vi "FFT_DAS_GUI(2).vi"() -> ()   [LabVIEW 2010]
doc: "<b>LITVC - ?????????????????????</b>\n\nMeasures, graphs and logs the data from the LITVC cRIO Chassis. Samples 12 analog channels of raw at kilohertz speeds, and controls starting of test data runs, with triggered control of the appropriate solenoid valves . \n\nSystem scaling and other constants are loaded from the \"LITVC_CFG.TXT\" text file at startup. (The order of the lines must remain the same. ) The Operator must supply a data file path and name at startup. This defaults on the cRIO Controller to: \"C:\\Data\". The software then starts data acquisition and logging, as indicated by the blinking green \"Active\" LED.\n\nPressing \"CAL\" after start will calibrate the system to the cross section of the wire rope.\nTo stop the acquisition, press the Stop button in the upper right. This allows the operator to look at the graphs, error indicators, etc on the status tab.\nTo Exit, press the EXIT button on the Status tab.\n\nVersion 1.0.0:\n 1. Initial version\n\n2010_09_30 Michael Ashe\nmichael.ashe@aztera.com\nmichael.ashe@imaginatics.net\n(860) 961-0876 (Cell)"
uses:
  Common/Controls/GUI_Buttons_23x22_W2K.llb/FileGroup_1.ctl
  Common/Controls/GUI_Buttons_23x22_W2K.llb/New.ctl
  Common/Controls/GUI_Buttons_23x22_W2K.llb/Open.ctl
  Common/Controls/GUI_Buttons_23x22_W2K.llb/Save.ctl
  Common/Controls/GUI_Buttons_23x22_W2K.llb/EditGroup_1.ctl
  Common/Controls/GUI_Buttons_23x22_W2K.llb/Cut.ctl
  Common/Controls/GUI_Buttons_23x22_W2K.llb/Copy.ctl
  Common/Controls/GUI_Buttons_23x22_W2K.llb/Paste.ctl
  Common/Controls/GUI_Buttons_23x22_W2K.llb/Delete1.ctl
  Common/Controls/GUI_Buttons_23x22_W2K.llb/MacroPlay.ctl
  Common/Controls/GUI_Buttons_23x22_W2K.llb/MacroPause.ctl
  Common/Controls/GUI_Buttons_23x22_W2K.llb/MacroStop.ctl
  Common/Controls/BlockStart Button.ctl
  Common/Controls/BlockEnd Button.ctl
  Common/Controls/Gauge TDef.ctl
  Common/Controls/Timing Mode.ctl
  Common/Module Manager/MM_Module_Control_Mode.ctl
  Common/GUI/Enable Controls API.llb/Action.ctl
  Common/StateFile.llb/Actions.ctl
  Common/Timing/Controls/StateMachineStates_TEST_TDEF.ctl
  Common/Module Manager/MM_Module_Action.ctl
  Common/COMM_Queues/Command_Queue_Select.ctl
  Common/COMM_Queues/Command Queue Cluster.ctl
  Common/Timing/Controls/Timer Actions ENUM_TEST_TDef.ctl
  Common/Globals/FFT_DAS-Editing Variables_GBL.vi
  <vilib>/Utility/file.llb/Read From Spreadsheet File (string).vi
  Instance           2 15Saved   WRIS_9g .vi
  <vilib>/Utility/file.llb/Write To Spreadsheet File (string).vi
  Common/GUI/Enable Controls.lvlib
panel:
  out "Current within Tolerance":bool
  out "Login Mode Out":enum32{"Editor", "Operator"}(ring)
  out "Diff. Press within Tolerance":bool
  out "Flow Meter":bool
  out "Thermocouple":bool
  out "Agilent":bool
  out "DAQ":bool
  in  "Rest All IO":bool
  in  "Exit":bool
  in  "Tab Control":enum32{"Test Run", "Report ", "Graphs", "Setup"}(tab)
  in  "Delete Config":T1
  in  "Go to Next Step":bool
  in  "BP Regulator Manual Control":bool
  in  "Current Manual Control":bool caption="Current Enabled"
  in  "Current Configration File":u16(ring)
  out "Actual  Voltage":dbl(slide) scale=0.0..20.0 scale format="%#_g V"
  out "Actual Current":dbl(slide) scale=0.0..360.0 scale format="%#_g mA"
  in  "Control Devices":cluster{"Current":dbl, "BP Regulator":dbl} {"BP Regulator" scale=0.0..100.0 scale format="%#3.2f%"; "Current" scale=0.0..300.0 scale format="%#_g mA"}
  out "Test Status":T2(ring)
  out "Analog Sensors":T3 {"Fuel Temp" scale=0.0..200.0 scale format="%#.1f °F"; "Flow" scale=0.0..1000.0; "Unused" scale=0.0..10.0; "Diff. Pressure (100psid)" scale=0.0..400.0; "Bypass Pressure" scale=0.0..200.0; "Back Pressure" scale=0.0..300.0; "Diff. Pressure  (50 psid)" scale=0.0..400.0; "Supply Pressure" scale=0.0..400.0}
  in  "BlkMrkGrp":cluster{"Block Start":T4, "Block End":T5}
  in  "MacroGroup":T9
  in  "Delete":T1
  in  "EditGroup_1":T10
  in  "FileGroup_1":T14
  in  "Test Table":string[][](table)=[["", "20", "10", "109 ", "200", " ", " ", " ", " ", " ", " ", " ", " ", " ", " "], ["", "40", "22", "160", "200", "", " ", " ", " ", " ", " ", " ", " ", " ", " "], ["", "10", "32", "400", "500", "", " ", " ", " ", " ", " ", " ", " ", " ", " "]] caption="A/M    Current      Dwell            Min Flow       Max Flow       Actual Flow    Hysteresis"
  out "EditLine":i32=65534
  out "EditCol":i32=65534
  in  "StartTest":bool
  in  "StopTest":bool
  in  "PauseTest":bool
  out "CountDown Pie":picture
  out "CountDown Text":string="0:00"
  in  "Test Timing Mode":T18
  in  "Config Actions":T14
  in  "Send to Excel":bool
  in  "Additional Report Values":cluster{"Excel  Name":string, "Value":string}[](array[cluster])
  out "Test Table2":string[][](table)=[["", "20", "10", "109 ", "200", " ", " ", " ", " ", " ", " ", " ", " ", " ", " "], ["", "40", "22", "160", "200", "", " ", " ", " ", " ", " ", " ", " ", " ", " "], ["", "10", "32", "400", "500", "", " ", " ", " ", " ", " ", " ", " ", " ", " "]] caption="Table"
  out "Parameter Table Out":string[][](table)
  out "Flow-Current XY Graph":cluster{cluster{"X":dbl, "Y":dbl}[]}[](graph)
  in  "Stability Dwell Time (sec)":dbl=50.0
  in  "Save Password":bool
  in  "Editor Password":string
  in  "Tolerance (psid)":dbl=50.0
  in  "reset":bool
  in  "Send PID":bool
  in  "System Refresh Button":bool
  in  "Enable":bool
  in  "Temp Channel":refnum<k21>="Fuel_Temp"
  in  "BP Regulator Command":refnum<k21>="BP_Regulator_Command"
  in  "Setpoint (psid)":dbl=50.0
  in  "Agilent Resource Name":refnum<visa-resource-name>="USB0::0x0957::0x4118::MY48130014::INSTR"
  in  "FEM-03 Port":refnum<visa-resource-name>="COM1"
  in  "Simulate Hardware":bool=TRUE
  out "USB 6211":errorcluster
  out "USB Agilent":errorcluster
  out "USB TC 01":errorcluster
  out "FEM-03":errorcluster
  out "Parameter Table Out 2":string[][](table) caption="Parameter Table + Comment Out"
  in  "Alarms":T19={"Flow"=0.0, "Flow 2"=0.0, "Fuel Temp"=350.0, "Fuel Temp 2"=0.0, "Supply Pressure"=250.0, "Supply Pressure "=200.0, "Diff. Pressure (50psid)"=100.0, "Diff. Pressure (50psid) 2"=20.0, "Back Pressure"=100.0, "Back Pressure 2"=20.0, "Bypass Pressure"=100.0, "Bypass Pressure 2"=20.0, "Diff. Pressure (100psid)"=100.0, "Diff. Pressure (100psid) 2"=20.0, "BP (Monitor)"=0.0, "BP (Monitor) 2"=0.0}
  out "Configuration Storage File":path
  in  "DAQ Channels":T20={"Supply Pressure"="Supply_Pressure_PX409", "DIff Pressure (50 psid)"="Diff_Pressure_2_D629", "Bypass pressure"="Bypass_Pressure_PX209", "Diff Pressure (100 psid)"="Diff_Pressure_1151", "BP Monitor"="BP-Monitor"}
  # "[n + offset]"
  # "-----Test Parameter Rows-------\n0-Step ID\n1-Current\n2-Dwell\n3-Min Flow\n4-Max Flow\n5-Hysteresis\n\n----TestData Rows---------\n6-Flow Rate\n7-Actual mA\n8-Temperature\nDAQ Sensor 1\nDAQ Sensor 2\nDAQ Sensor 3\n.\n.\nDAQ Sensor N"
  # "Sensor Alarms"
  # "External Instruments"
  # "Control Parameters"
  # "DAQ Channels"
  # "Differential \n-----------------------------------------------------------"
  # "Advanced Settings"
  # "LO Alarm"
  # "HI Alarm"
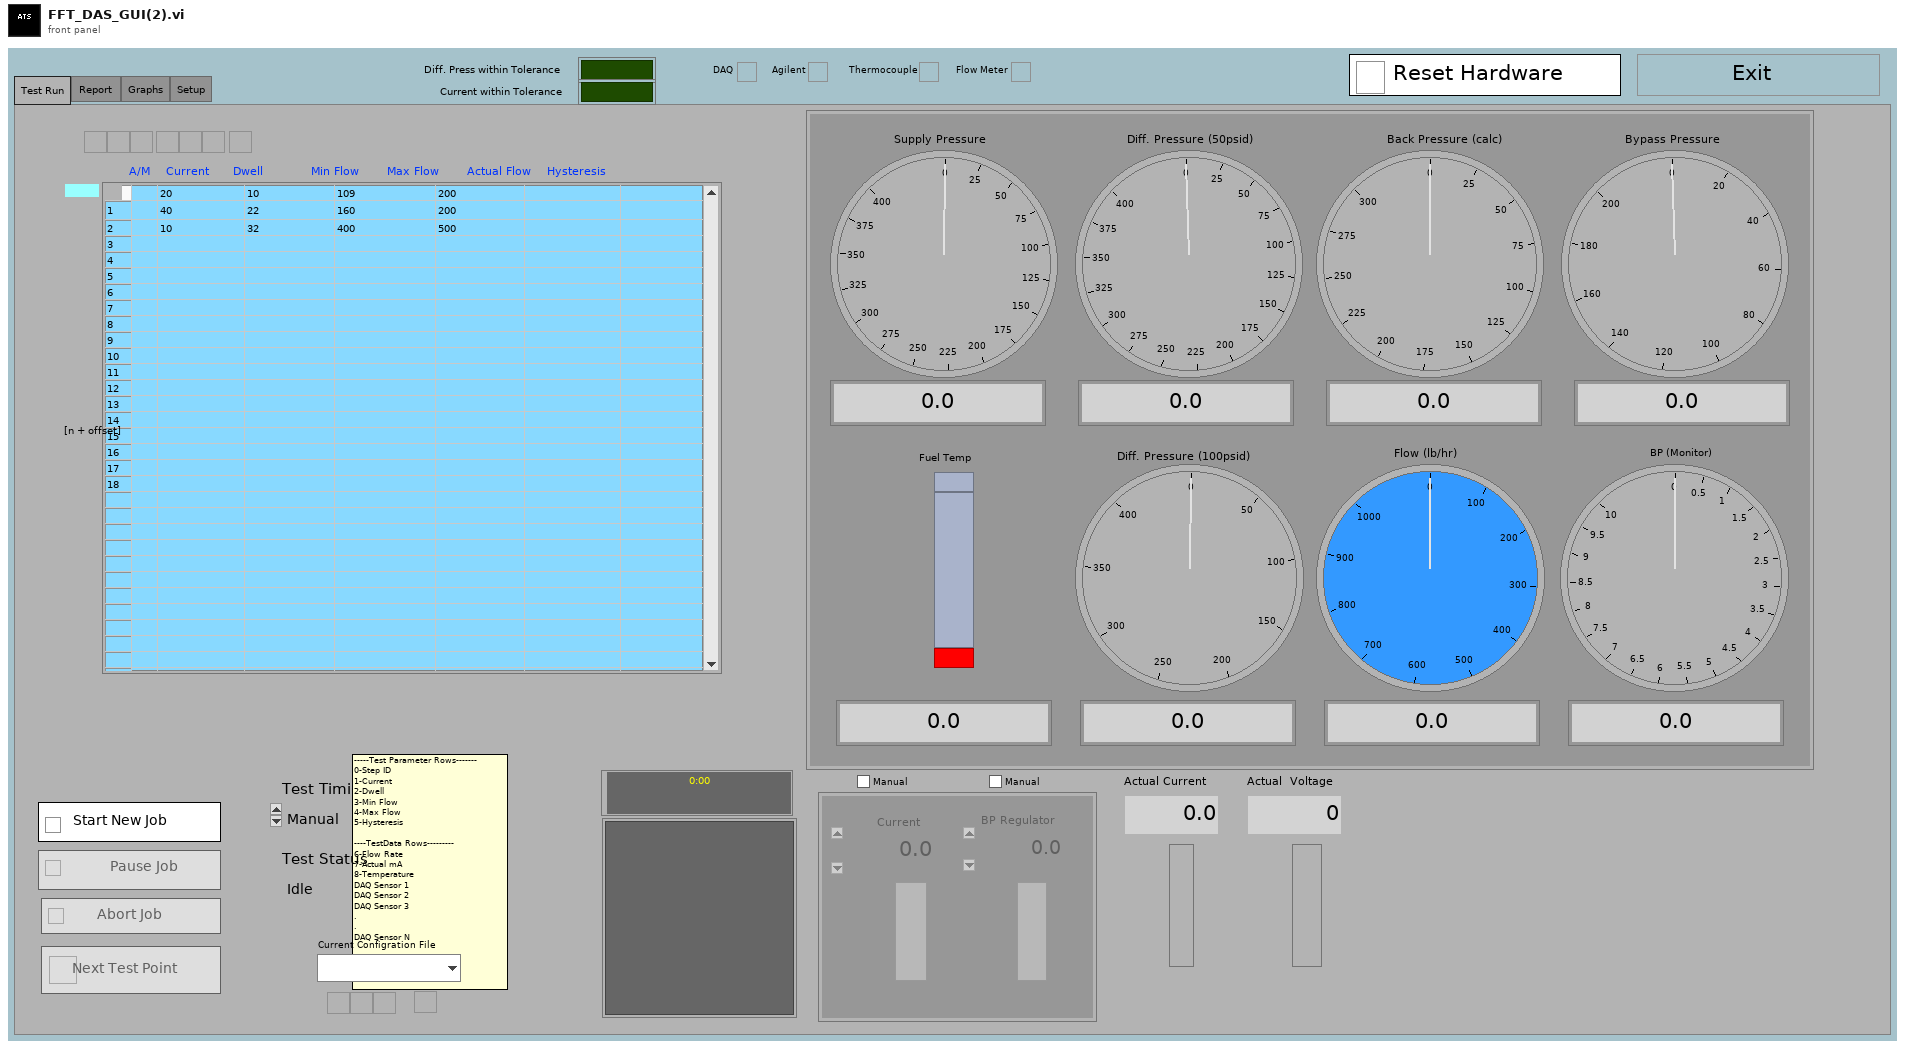
[diagram p1: front panel]
types:
  T1 = typedef "Delete1.ctl" = bool
  T2 = enum16{"Idle", "Test Running", "Test Paused", "Test Completed"}
  T3 = typedef "Gauge TDef.ctl" = cluster{"Flow":dbl, "Fuel Temp":dbl, "Supply Pressure":dbl, "Diff. Pressure  (50 psid)":dbl, "Back Pressure":dbl, "Bypass Pressure":dbl, "Diff. Pressure (100psid)":dbl, "Unused":dbl}
  T4 = typedef "BlockStart Button.ctl" = bool
  T5 = typedef "BlockEnd Button.ctl" = bool
  T6 = typedef "MacroPlay.ctl" = bool
  T7 = typedef "MacroPause.ctl" = bool
  T8 = typedef "MacroStop.ctl" = bool
  T9 = cluster{"MacroPlay":T6, "MacroPause":T7, "MacroStop":T8, "MacroName":u16}
  T10 = typedef "EditGroup_1.ctl" = cluster{"Cut":T11, "Copy":T12, "Paste":T13}
  T11 = typedef "Cut.ctl" = bool
  T12 = typedef "Copy.ctl" = bool
  T13 = typedef "Paste.ctl" = bool
  T14 = typedef "FileGroup_1.ctl" = cluster{"New":T15, "Open":T16, "Save":T17}
  T15 = typedef "New.ctl" = bool
  T16 = typedef "Open.ctl" = bool
  T17 = typedef "Save.ctl" = bool
  T18 = typedef "Timing Mode.ctl" = enum16{"Manual", "Automatic", "Semi-Automatic"}
  T19 = cluster{"Flow":dbl, "Flow 2":dbl, "Fuel Temp":dbl, "Fuel Temp 2":dbl, "Supply Pressure":dbl, "Supply Pressure ":dbl, "Diff. Pressure (50psid)":dbl, "Diff. Pressure (50psid) 2":dbl, "Back Pressure":dbl, "Back Pressure 2":dbl, "Bypass Pressure":dbl, "Bypass Pressure 2":dbl, "Diff. Pressure (100psid)":dbl, "Diff. Pressure (100psid) 2":dbl, "BP (Monitor)":dbl, "BP (Monitor) 2":dbl}
  T20 = cluster{"Supply Pressure":refnum<k21>, "DIff Pressure (50 psid)":refnum<k21>, "Bypass pressure":refnum<k21>, "Diff Pressure (100 psid)":refnum<k21>, "BP Monitor":refnum<k21>}
  T21 = typedef "Enable Controls.lvlib/Action.ctl" = enum16{"Editor Init", "Init", "Operator Init", "Timed Test Start", "Manual Test Start", "Stop Test", "Close", "Set States"}
  T22 = cluster{"Additional Parameter Section":string, "Blowfish Master Password":string, "Key Name":string, "Use Encryption":bool}
  T23 = typedef "Actions.ctl" = enum16{"Initialize", "Save VI State", "Load VI State", "Delete State", "Get All VI State Names", "Clear All States", "Close Global State File", "Open State File", "Create State File", "Write Data to File", "Exit"}
  T24 = enum16{"get data", "set data", "Add Data Pair", "initialize"}
  T25 = enum16{"get data", "set manual data", "set automatic data", "Set Mode", "initialize"}
  T26 = enum16{"Init", "Add Alarm Limits", "Update Flow Limit", "Check for Alarm", "Clear Alarms"}
  T27 = typedef "StateMachineStates_TEST_TDEF.ctl" = enum16{"Initialize", "Start", "Run Position", "Pause", "Resume", "Get Step", "Force Next Step", "Stay on Current Step"}
  T28 = typedef "MM_Module_Control_Mode.ctl" = enum16{"Get", "Set", "Init", "Get Initial Modules", "Add"}
  T29 = typedef "Internal State Data.ctl" = cluster{"StateFile Reference":T30, "StateFile Filepath":path, "Error":errorcluster, "VI ":enum16{"By VI Name", "Calling VI"}, "VI Name":string, "State":enum16{"By State Name", "Default State"}, "State Name":string, "notifier in":refnum<notifier>, " Progress Bar":bool}
  T30 = typedef "NI_LVConfig.lvlib/Config Data RefNum.ctl" = refnum<k1>
  T31 = typedef "FFT_DAS Shift Variables.ctl" = cluster{"queue data":T32, "error":errorcluster, "FFT_DAS queue":T33, "Q_TO":i32, "WDT_TO":dbl, "LogErrors?":bool, "Main.ini Ref":refnum<k1>, "Connected? 1":bool, "Address 1":string, "Link_Name":string, "Config Vars":T34, "DataFilePath":path, "Calibrate":bool, "Cal_Slope-Offset":dbl[][], "TestTable":string[][], "Test Status":enum16{"Idle", "Test Running", "Test Paused", "Test Completed"}, "Parameter Table Out":string[][], "Test Start Time":string, "Test Stop Time":string, "Test Timing Mode":T18, "Login Mode":enum32{"Editor", "Operator"}, "Editor Password":string, "Number of sensors":dbl}
  T32 = typedef "Command Queue Cluster.ctl" = cluster{"Command":string, "Variant Data":variant}
  T33 = typedef "Command_Queue_Ref.ctl" = refnum<queue>
  T34 = typedef "WRIS_Config Vars Cluster.ctl" = cluster{"Distance/Count":dbl, "samples/ch":i32, "Task_TO":dbl, "Kc":dbl, "B":dbl}
  T35 = typedef "MM_Module_Action.ctl" = enum16{"Idle", "Start", "Run", "Exit"}
  T36 = enum16{"STARTUP", "ERROR", "OPEN", "CLOSE", "ENABLE", "DISABLE", "SHUTDOWN"}
  T37 = typedef "Command_Queue_Select.ctl" = enum16{"<no op>", "Destroy Queues", "Send -> State_Machine", "Send -> Client_IO", "Send -> Logging", "Send -> Instrument_IO", "Send -> Tag_Manager", "Send -> Alarms_Shutdowns", "Send -> Control_Loops", "Send -> Server_IO", "Send -> GUI"}
  T38 = enum8{"Enabled", "Disabled", "Disabled and Grayed Out"}
  T39 = enum16{"Init", "Add Alarm Limits", "Update Flow Limit", "Check for Alarm", "Clear Alarms", "Set Enable Status"}
  T40 = enum16{"get data", "set raw data", "Set Ti and SGi and SGH20", "Add New Formula", "Get Formula", "initialize"}
  T41 = cluster{"State":enum16{"By State Name", "Default State"}, "State Name":string}
  T42 = cluster{"Flow Calibration Formula":string, "Valid Flow Ranges":dbl[]}[]
  T43 = cluster{"Temp  Out":dbl, "Specific Gravity Out":dbl}
  T44 = cluster{"[0]":dbl, "[1]":dbl, "[2]":dbl, "[3]":dbl, "[4]":dbl, "[5]":dbl, "[6]":dbl, "[7]":dbl}
  T45 = cluster{"Flow Calibration Formula":string, "Specific Gravity Calibration Formula":string, "Flow Conversion Formula":string}
  T46 = typedef "Timer Actions ENUM_TEST_TDef.ctl" = enum16{"Set Time", "Get Time", "Pause Time", "Resume Time"}
  T47 = typedef "LVRowAndColumnTypeDef.ctl" = cluster{"Row":i32, "Column":i32}
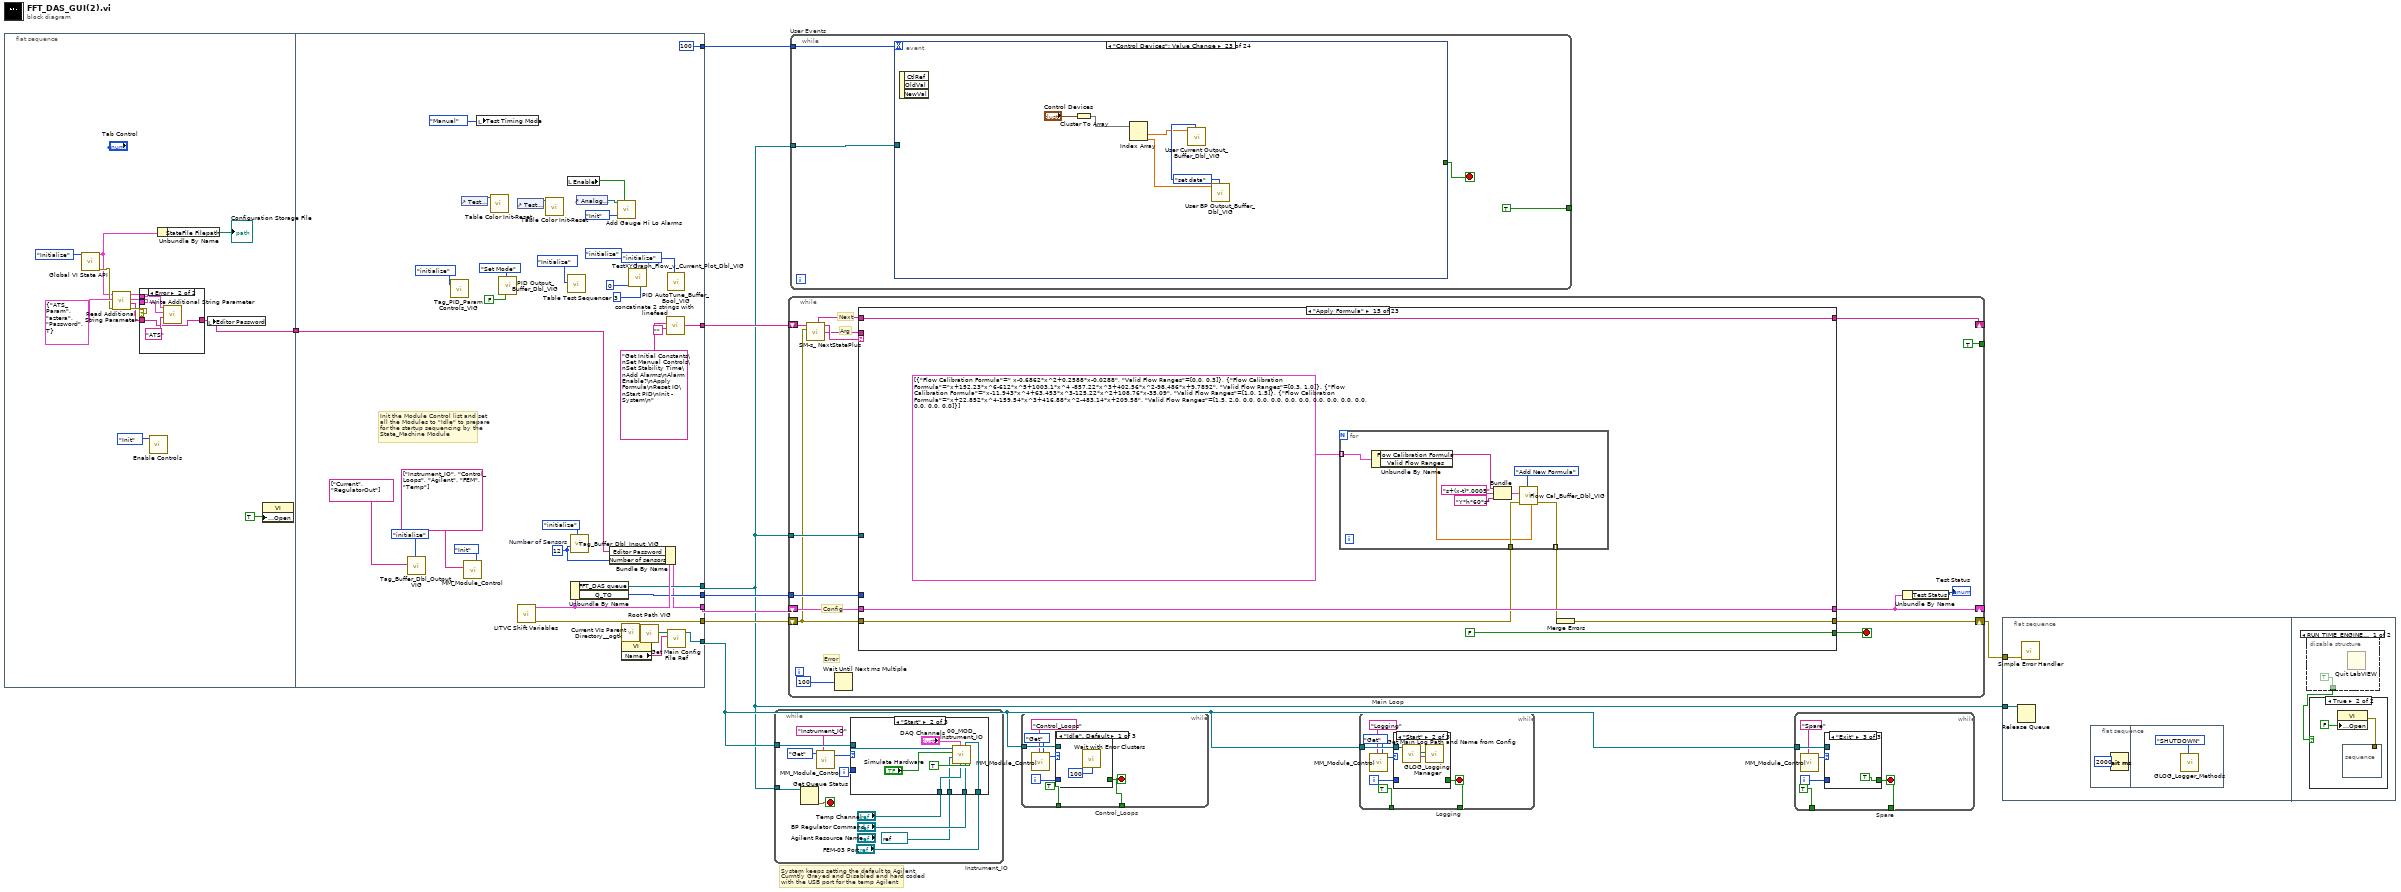
[diagram p0: block diagram]
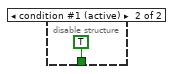
[diagram p2: hidden frame]
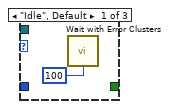
[diagram p5: hidden frame]
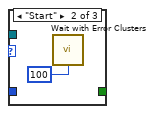
[diagram p6: hidden frame]
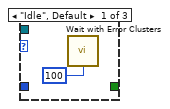
[diagram p7: hidden frame]
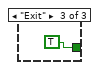
[diagram p8: hidden frame]
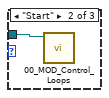
[diagram p9: hidden frame]
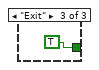
[diagram p10: hidden frame]
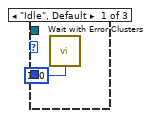
[diagram p11: hidden frame]
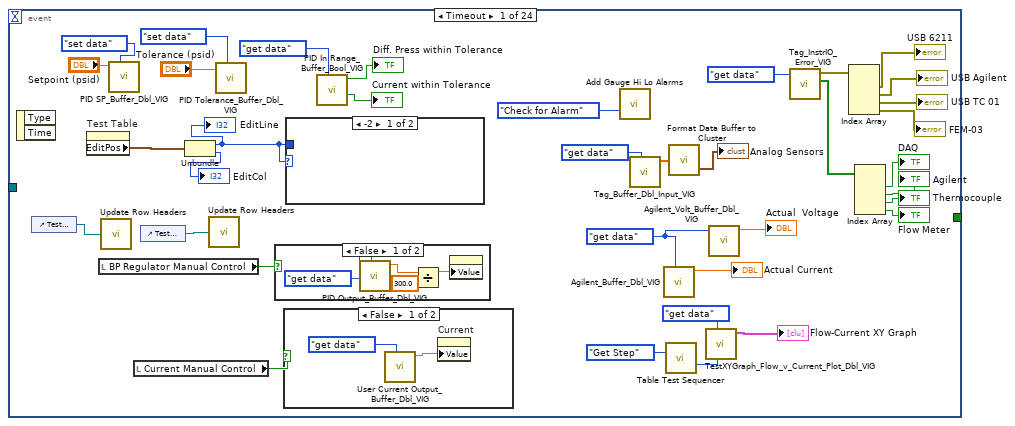
[diagram p13: hidden frame]
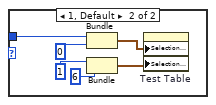
[diagram p16: hidden frame]
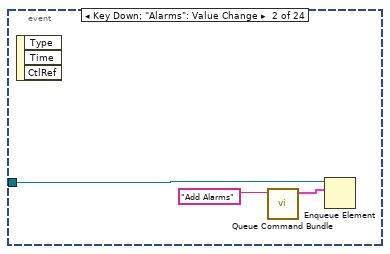
[diagram p17: hidden frame]
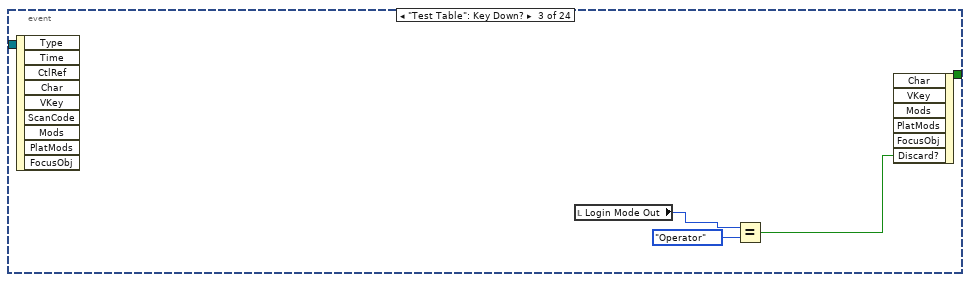
[diagram p18: hidden frame]
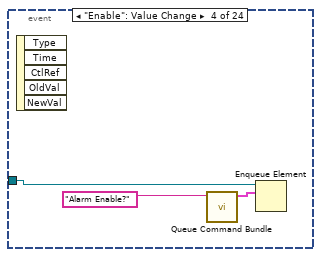
[diagram p19: hidden frame]
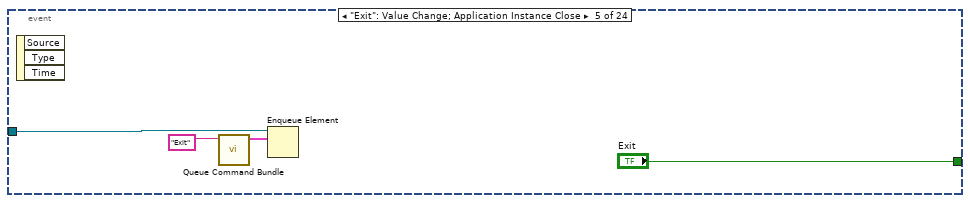
[diagram p20: hidden frame]
diagram:
  # "System keeps setting the default to Agilent\nCurrntly Grayed and Disabled and hard coded\nwith the USB port for the temp Agilent"
  n1 = flat-sequence {
    tunnel: [w13] -> w1
    tunnel: [w59] -> w7
    tunnel: [w56] -> w8
    tunnel: [100] -> w6
    tunnel: [w30] -> w5
    tunnel: [w54] -> w4
    tunnel: [w53] -> w2
    tunnel: [w51] -> w3
    tunnel: w1 -> [w28]
    frame #0 {
      n2 = call "Global VI State API.vi"("Action"=Actions."Initialize") -> ("Internal State Data"=w11:T29, "Error"=w16:errorcluster)  [unwired: 12 in, 1 out]
      n3 = call "Read Additional String Parameter.vi"("error in (no error)"=w16, "Additional Parameters Out"=T22 {"Additional Parameter Section"="ATS_Param", "Blowfish Master Password"="aztera", "Key Name"="Password", "Use Encryption"=TRUE}, "Internal State Data"=w11) -> ("error out"=w19:errorcluster, "Value"=w15:string, "Additional Parameters Out"=w17:T22, "Internal State Data  Out"=w18:T29)  [unwired: 5 in]
      n4 = case shown="Error" w19 {
        tunnel: w18 -> [_ w26]
        tunnel: w17 -> [_ w25]
        tunnel: w15 -> [w22 w23]
        tunnel: [w22 w23] -> w13
        frame No Error {
        }
        frame Error {
          n5 = call "Write Additional String Parameter.vi"("value"="ATS", "Additional Parameters Out"=w25, "Internal State Data"=w26) -> ()  [unwired: 6 in, 3 out]
        }
      }
      n6 = call "Enable Controls.vi"("Enabled State"=Action."Init") -> ()  [unwired: 10 in, 1 out]
      n7 = Unbundle By Name(w11) -> ("StateFile Filepath"=→"Configuration Storage File":path)
      n8 = local write "Editor Password"(w13) -> ()
      n9 = property class="VI"("Front Panel.Open"=TRUE) -> ()  [unwired: 2 in, 2 out]
    }
    frame #1 {
      w29 = 12  # Number of Sensors
      # "Init the Module Control list and set\nall the Modules to \"Idle\" to prepare\nfor the startup sequencing by the\nState_Machine Module"
      n10 = call "Tag_Buffer_Dbl_Output_VIG.vi"("Operation"=enum16{"get data", "set data", "initialize"}."initialize", "tag_names_in"=string[] ["Current", "RegulatorOut"]) -> ()  [unwired: 7 in, 3 out]
      n11 = call "Tag_PID_Param Controls_VIG.vi"("Operation"=enum16{"get data", "set data", "initialize"}."initialize") -> ()  [unwired: 9 in, 2 out]
      n12 = control-ref of="Test Table2"() -> (w36:refnum<vi>)
      n13 = call "MM_Module_Control.vi"("MM_Module_Ctrlr_Mode"=MM_Module_Control_Mode."Init", "Module_Names_Initial"=string[] ["Instrument_IO", "Control_Loops", "Agilent", "FEM", "Temp"] ("Column Header Strings[]")) -> ()  [unwired: 6 in, 4 out]
      n14 = local write "Test Timing Mode"(Timing_Mode."Manual" ("Test Timing Mode")) -> ()
      n15 = call "Table Color Init-Reset.vi"("Test Table"=w36) -> ()  [unwired: 11 in]
      n16 = call "PID Output_Buffer_Dbl_VIG.vi"("Automatic"=FALSE, "Operation"=T25."Set Mode") -> ()  [unwired: 8 in, 2 out]
      n17 = control-ref of="Test Table"() -> (w45:refnum<vi>)
      n18 = call "LITVC Shift Variables.vi"() -> ("error out"=w56:errorcluster, "VARS FFT_DAS"=w55:T31)  [unwired: 10 in]
      n19 = call "Table Color Init-Reset.vi"("Test Table"=w45) -> ()  [unwired: 11 in]
      n20 = local read "Enable"() -> (w40:bool)
      n21 = call "Table Test Sequencer.vi"("Action"=StateMachineStates_TEST_TDEF."Initialize") -> ()  [unwired: 3 in, 8 out]
      n22 = call "Tag_Buffer_Dbl_Input_VIG.vi"("Operation"=enum16{"get data", "set data", "initialize"}."initialize", "Number of Sensors"=w29) -> ()  [unwired: 8 in, 2 out]
      n23 = Unbundle By Name(w55) -> ("FFT_DAS queue"=w53:T33, "Q_TO"=w54:i32)
      n24 = control-ref of="Analog Sensors"() -> (w44:refnum<vi>)
      n25 = Bundle By Name(cluster=w55, "Editor Password"=w28, "Number of sensors"=w29) -> (w30:T31)
      n26 = call "Add Gauge Hi Lo Alarms.vi"("Enable"=w40, "Action"=T26."Init", "reference"=w44) -> ()  [unwired: 8 in]
      n27 = call <userlib>:"Current VIs Parent Directory__ogtk.vi"() -> ("Parent Directory (+ Relative)"=w49:path)  [unwired: 5 in]
      n28 = property class="VI"() -> ("Name"=w52:string)  [unwired: 2 in, 2 out]
      n29 = call "TestXYGraph_Flow_v_Current_Plot_Dbl_VIG.vi"("Plot Index/Size"=3, "Point index/size"=0, "Operation"=T24."initialize") -> ()  [unwired: 6 in, 3 out]
      n30 = call "Root Path VIG.vi"("Set Root VI's Path"=w49) -> ("Root VI's Path"=w48:path)
      n31 = call "concatinate 2 strings with linefeed.vi"("String 2"="", "String 1"="Get Initial Constants\nSet Manual Controls\nSet Stability Time\nAdd Alarms\nAlarm Enable?\nApply Formula\nReset IO\nStart PID\nInit - System\n") -> ("Concatinated OUT"=w59:string)  [unwired: 6 in]
      n32 = call "PID AutoTune_Buffer_Bool_VIG.vi"("Operation"=enum16{"get data", "set data", "initialize"}."initialize") -> ()  [unwired: 9 in, 2 out]
      n33 = call "Get Main Config File Ref.vi"("Main VI Name"=w52, "Main VI Directory"=w48) -> ("Main Config File Refnum"=w51:T30)  [unwired: 8 in, 1 out]
    }
  }
  n34 = while "Instrument_IO" {
    tunnel: w3 -> [w69]
    tunnel: w2 -> [w66]
    i -> [w70]
    stop <- w67 stop-if-true
    n35 = Get Queue Status(queue=w66) -> (error out=w67:errorcluster)  [unwired: 2 in, 7 out]
    n36 = call "MM_Module_Control.vi"("MM_Module_Ctrlr_Mode"=MM_Module_Control_Mode."Get", "Module Name"="Instrument_IO") -> ("MM_Module_Action Out"=w71:T35)  [unwired: 6 in, 3 out]
    n37 = case shown="\"Start\"" w71 {
      tunnel: w70 -> [_ _ _]
      tunnel: w69 -> [_ w80 _]
      tunnel: "FEM-03 Port" -> [_ w77 _]
      tunnel: "BP Regulator Command" -> [_ w76 _]
      tunnel: "Temp Channel" -> [_ w75 _]
      tunnel: refnum<visa-resource-name> "USB0::0x0957::0x4118::MY51200023::INSTR" ("Agilent Resource Name") -> [_ w74 _]
      frame "Idle", Default {
        n38 = call "Wait with Error Clusters.vi"("Wait (mS)"=u32 100 ("Milliseconds to Wait (500)")) -> ()  [unwired: 14 in, 1 out]
      }
      frame "Start" {
        n39 = call "00_MOD_Instrument_IO.vi"("AI Averaging On"=TRUE, "BP Regulator Channel"=w76, "FEM"=w77, "Temp Channel"=w75, "DAQ Sensor Channels"="DAQ Channels", "Agilent"=w74, "Simulate"="Simulate Hardware", "Main Config File Refnum"=w80) -> ()  [unwired: 3 in, 1 out]
      }
      frame "Exit" {
      }
    }
  }
  n40 = while "Main Loop" {
    shift-right: [w94] -> _
    shift-left: w7 -> [w85]
    shift-right: [w84] -> _
    shift-left: w5 -> [w95]
    shift-right: [w81] -> w9
    shift-left: w8 -> [w86]
    tunnel: w4 -> [w88]
    tunnel: w2 -> [w87]
    tunnel: [TRUE] -> _
    stop <- w89 stop-if-true
    # "Arg"
    # "Next"
    # "Error"
    # "Config"
    n41 = call "SM-s_ NextStatePlus.vi"("error?"=w86, "States String"=w85) -> ("Argument"=w92:string, "Current State"=w93:string, "Next States"=w91:string)  [unwired: 7 in]
    n42 = Wait Until Next ms Multiple(millisecond multiple=u32 100 ("Loop Wait (mSec)")) -> ()  [unwired: 1 out]
    n43 = case shown="\"Apply Formula\"" w93 {
      tunnel: w95 -> [w96 w190 w196 w206 w212 w226 w232 w243 w283 w308 w326 w330 w333 w352 w377 w390 w425 w432 w436 w453 w514 w518 w530]
      tunnel: [w104 w190 w196 w206 w212 w226 w232 w243 w286 w312 w326 w330 w332 w352 w377 w404 w424 w431 w442 w477 w514 w518 w530] -> w84
      tunnel: w86 -> [w101 w187 w191 w203 w209 w223 w227 w239 w281 w309 w315 w327 w334 w348 w374 w388 w420 w427 w434 w472 w511 w516 w525]
      tunnel: [w97 w187 w191 w203 w209 w223 w227 w239 w266 w309 w315 w327 w334 w348 w371 w388 w420 w427 w434 w472 w511 w516 w525] -> w81
      tunnel: [w99 w189 w197 w205 w211 w225 w231 w242 w288 w310 w325 w329 w336 w351 w376 w401 w421 w428 w438 "Check CmdQ" ("Next States") w513 w517 w531] -> w94
      tunnel: w92 -> [_ _ _ _ _ _ _ _ _ _ _ _ _ _ _ _ _ _ _ _ _ _ w529]
      tunnel: w91 -> [w100 w189 w197 w205 w211 w225 w231 w242 w288 w310 w325 w329 w336 w351 w376 w402 w421 w428 w438 _ w513 w517 w531]
      tunnel: [FALSE TRUE TRUE FALSE FALSE FALSE FALSE FALSE FALSE FALSE FALSE FALSE FALSE FALSE FALSE FALSE FALSE FALSE FALSE FALSE FALSE _ FALSE] -> w89
      tunnel: w88 -> [w106 _ _ _ _ _ _ _ _ _ _ _ _ _ _ _ _ _ _ _ _ _ _]
      tunnel: w87 -> [w105 _ _ _ _ _ _ _ _ _ _ _ _ _ _ _ _ _ _ _ _ _ _]
      frame "Check CmdQ", Default {
        # "NOTE: The timeout might need to be\nadjusted if the data read rate changes\nso that we needed to read more often\nthan 100x sec      (unlikely)."
        # "incoming Cmd"
        # "Push incomming command\nto top of command stack"
        # "Quick check if there is\na new command, if not\ngo back to \"Get Data\""
        n44 = call "Queue Command Read & Parse.vi"("Q_TO"=w106, "Command_Q"=w105) -> ("Variant Data"=w103:variant, "Command"=w102:string)  [unwired: 6 in, 2 out]
        n45 = case shown="\"Change Timing Mode\"" w102 {
          selector: w102 -> [w111 _ _ _]
          tunnel: w96 -> [w108 w130 w143 w185]
          tunnel: [w108 w130 w143 w186] -> w104
          tunnel: w103 -> [_ _ w139 w184]
          tunnel: [w115 "Exit" w146 _] -> w98
          tunnel: w101 -> [w117 w121 w138 w181]
          tunnel: [w117 w121 w135 w181] -> w97
          frame "Q_Timeout", Default {
            n46 = Unbundle By Name(w108) -> ("Test Status"=w116:T2)
            n47 = Equal?(x=w111, y="Q_Timeout") -> (x = y?=w112:bool)
            n48 = Select(t="", s=w112, f=w111) -> (s? t:f=w110:string)
            n49 = case shown="\"Test Running\"" w116 {
              tunnel: ["" ("element") "Run Test" ("element") "Stop Test\nSend to Excel\nSet Status to Idle" ("element")] -> w114
              frame "Idle", Default {
              }
              frame "Test Running" {
              }
              frame "Test Completed" {
              }
            }
            n50 = call "concatinate 2 strings with linefeed.vi"("String 2"=w114, "String 1"=w110) -> ("Concatinated OUT"=w115:string)  [unwired: 6 in]
          }
          frame "Exit" {
            n51 = for {
              tunnel: MM_Module_Control_Mode."Set" ("MM_Module_Ctrlr_Mode") -> [w134]
              tunnel: MM_Module_Action."Exit" ("MM_Module_Action In") -> [w133]
              tunnel: string[] ["GUI_IO", "Logging"] ("Module_Names_Initial") -> [w132] mode=indexing
              tunnel: [w131] -> w122
              n52 = call "MM_Module_Control.vi"("MM_Module_Ctrlr_Mode"=w134, "Module Name"=w132, "MM_Module_Action In"=w133) -> ("error out"=w131:errorcluster)  [unwired: 5 in, 3 out]
            }
            n53 = call "API Queue Manager.vi"("Q_Select"=Command_Queue_Select."Send -> Client_IO", "error in (no error)"=w122, "Command"="shutdown") -> ()  [unwired: 7 in, 2 out]
            n54 = call "GLOG_Logger_Methods.vi"("Logger Method"=T36."SHUTDOWN", "error in (no error)"=w122) -> ()  [unwired: 8 in, 2 out]
          }
          frame "ReceiveCMD" {
            # "This will be filled in with commands to\nStartTest:FileNamePath\nStopTest\nCalibrate"
            n55 = Variant To Data(error in=w138, Variant=w139, type="") -> (error out=w140:errorcluster, data=w142:string)
            n56 = Unflatten From String(type=T32 {"Command"="", "Variant Data"=variant} ("queue data"), binary string=w142, error in (no error)=w140) -> (value=w136:T32, error out=w135:errorcluster)  [unwired: 2 in, 1 out]
            n57 = Unbundle By Name(w136) -> ("Command"=w145:string, "Variant Data"=w144:variant)
            n58 = case shown="\"ListDataFiles\"" w145 {
              selector: w145 -> [_ w148 w153 w156 _ _]
              tunnel: ["Error Handle" ("element") w148 w153 w156 "" ""] -> w146
              tunnel: w144 -> [_ _ w152 _ _ w171]
              frame "", Default {
              }
              frame "Calibrate" {
              }
              frame "Init - Datalog" {
                n59 = Variant To Data(Variant=w152, type=path "") -> (error out=w150:errorcluster, data=w151:path)  [unwired: 1 in]
                n60 = call "WRIS_DataFilePath_VIG.vi"("Operation"=enum16{"get data", "set data"}."set data", "error in"=w150, "DataFilePath_in"=w151) -> ()  [unwired: 7 in, 2 out]
              }
              frame "Stop - Datalogging" {
                n61 = call "WRIS_DataFilePath_VIG.vi"("Operation"=enum16{"get data", "set data"}."set data", "DataFilePath_in"=path "") -> ()  [unwired: 8 in, 2 out]
              }
              frame "ListDataFiles" {
                n62 = call <userlib>:"Current VIs Parent Directory__ogtk.vi"("Relative path (.)"=path "Data files") -> ("Parent Directory (+ Relative)"=w164:path)  [unwired: 4 in]
                n63 = List Folder(path=w164) -> (filenames=w158:string[])  [unwired: 3 in, 3 out]
                n64 = call "Queue Command Bundle.vi"("Variant Data"=w158, "Command"="DataFileList" ("element")) -> ("main window queue datatype"=w160:T32)  [unwired: 9 in]
                n65 = To Variant(anything=w160) -> (Variant=w159:variant)
                n66 = call "API Queue Manager.vi"("Q_Select"=Command_Queue_Select."Send -> Client_IO", "Variant Data"=w159, "Command"="SendSTATUS") -> ()  [unwired: 7 in, 2 out]
              }
              frame "GetDataFile" {
                n67 = Variant To Data(Variant=w171, type="") -> (data=w170:string)  [unwired: 1 in, 1 out]
                n68 = call <userlib>:"Current VIs Parent Directory__ogtk.vi"("Relative path (.)"=path "Data files") -> ("Parent Directory (+ Relative)"=w173:path)  [unwired: 4 in]
                n69 = Build Path(base path=w173, name or relative path=w170) -> (appended path=w169:path)
                n70 = Read from Text File(file (use dialog)=w169, count=-1) -> (text=w168:string)  [unwired: 2 in, 3 out]
                n71 = call "Queue Command Bundle.vi"("Variant Data"=w168, "Command"="DataFile" ("element")) -> ("main window queue datatype"=w176:T32)  [unwired: 9 in]
                n72 = To Variant(anything=w176) -> (Variant=w175:variant)
                n73 = call "API Queue Manager.vi"("Q_Select"=Command_Queue_Select."Send -> Client_IO", "Variant Data"=w175, "Command"="SendSTATUS") -> ()  [unwired: 7 in, 2 out]
              }
            }
          }
          frame "Change Timing Mode" {
            n74 = Variant To Data(Variant=w184, type=Timing_Mode."Semi-Automatic" ("Test Timing Mode")) -> (data=w182:T18)  [unwired: 1 in, 1 out]
            n75 = Bundle By Name(cluster=w185, "Test Timing Mode"=w182) -> (w186:T31)
          }
        }
        n76 = call "concatinate 2 strings with linefeed.vi"("String 2"=w100, "String 1"=w98) -> ("Concatinated OUT"=w99:string)  [unwired: 6 in]
      }
      frame "Error Handle" {
      }
      frame "Exit" {
        n77 = for {
          tunnel: string[] ["Control", "Instrument_IO"] -> [w199] mode=indexing
          tunnel: [w198] -> w192
          n78 = call <vilib>:"Stop Timed Structure.vi"("name"=w199) -> ("error out"=w198:errorcluster)  [unwired: 10 in]
        }
        n79 = for {
          tunnel: string[] ["Logging", "Instrument_IO", "Control_Loops"] ("Column Header Strings[]") -> [w201] mode=indexing
          tunnel: w192 -> [_]
          n80 = call "MM_Module_Control.vi"("MM_Module_Ctrlr_Mode"=MM_Module_Control_Mode."Set", "Module Name"=w201, "MM_Module_Action In"=MM_Module_Action."Exit") -> ()  [unwired: 5 in, 4 out]
        }
      }
      frame "----- Initialization -----" {
        # "This case should never run\nIt is for State Machine organization only"
      }
      frame "Set Stability Time" {
        n81 = call "SP Stability_Buffer_Dbl_VIG.vi"("Operation"=enum16{"get data", "set data", "initialize"}."set data", "Time (sec)"="Stability Dwell Time (sec)") -> ()  [unwired: 8 in, 2 out]
      }
      frame "Set Manual Controls" {
        n82 = Select(t=T38."Enabled" ("Disabled"), s="BP Regulator Manual Control", f=T38."Disabled and Grayed Out" ("Disabled")) -> (s? t:f=w217:T38)
        n83 = Select(t=T38."Enabled" ("Disabled"), s="Current Manual Control", f=T38."Disabled and Grayed Out" ("Disabled")) -> (s? t:f=w213:T38)
        n84 = property on="BP Regulator" class="Slide (strict)"("DisabledEnum"=w217) -> ()  [unwired: 2 in, 2 out]
        n85 = Not(x="BP Regulator Manual Control") -> (.not. x?=w222:bool)
        n86 = property on="Current" class="Slide (strict)"("DisabledEnum"=w213) -> ()  [unwired: 2 in, 2 out]
        n87 = call "PID Output_Buffer_Dbl_VIG.vi"("Automatic"=w222, "Operation"=T25."Set Mode") -> ()  [unwired: 8 in, 2 out]
      }
      frame "Alarm Enable?" {
        n88 = call "Add Gauge Hi Lo Alarms.vi"("Enable"="Enable", "Action"=T39."Clear Alarms") -> ()  [unwired: 9 in]
      }
      frame "Reset IO" {
        n89 = call "IO Active_Buffer_Bool_VIG.vi"("Operation"=enum16{"get data", "set data", "initialize"}."set data", "Boolean"=FALSE) -> ("error out"=w237:errorcluster)  [unwired: 8 in, 1 out]
        n90 = for {
          tunnel: string[] ["Instrument_IO"] -> [w263] mode=indexing
          tunnel: [w262] -> w234
          tunnel: w237 -> [w261]
          n91 = call <vilib>:"Stop Timed Structure.vi"("error in (no error)"=w261, "name"=w263) -> ("error out"=w262:errorcluster)  [unwired: 9 in]
        }
        n92 = flat-sequence {
          tunnel: [w244] -> w233
          tunnel: w234 -> [_]
          frame #0 {
            n93 = call "MM_Module_Control.vi"("MM_Module_Ctrlr_Mode"=MM_Module_Control_Mode."Set", "Module Name"="Instrument_IO", "MM_Module_Action In"=MM_Module_Action."Start") -> ("error out"=w244:errorcluster)  [unwired: 5 in, 3 out]
          }
        }
        n94 = Tick Count (ms)() -> (millisecond timer value=w238:u32)
        n95 = while {
          tunnel: w238 -> [w256]
          tunnel: w233 -> [_]
          i -> [w252]
          stop <- w250 stop-if-true
          n96 = Wait (ms)(milliseconds to wait=u32 100) -> (millisecond timer value=w257:u32)
          n97 = Subtract(x=w257, y=w256) -> (x-y=w255:u32)
          n98 = call "IO Active_Buffer_Bool_VIG.vi"("Operation"=enum16{"get data", "set data", "initialize"}."get data", "Boolean"=FALSE) -> ("Boolean 2"=w258:bool)  [unwired: 8 in, 1 out]
          n99 = Greater?(x=w255, y=u32 60000 ("milliseconds to wait")) -> (0:w253:bool)
          n100 = Or(x=w253, y=w258) -> (x .or. y?=w251:bool)
          n101 = call "Progress.vi"("iteration"=w252, "Message"="Resetting IO....." ("String 2"), "Stop"=w251) -> ("stop"=w250:bool)  [unwired: 8 in]
        }
      }
      frame "Get Initial Constants" {
        n102 = call "Global VI State API.vi"("Action"=Actions."Get All VI State Names") -> ("VI States"=w273:string[])  [unwired: 12 in, 2 out]
        n103 = property on="Current Configration File" class="Ring (strict)"("Strings []"=w273) -> ()  [unwired: 2 in, 2 out]
        n104 = Unbundle By Name(w283) -> ("Editor Password"=w282:string)
        n105 = First Call?() -> (First Call?: T/F=w264:bool)
        n106 = call "Test Information Dialog.vi"("Part Numbers"=w273, "error in"=w281, "Editor Master Password"=w282, "Login Mode Input"=enum32{"Editor", "Operator"}."Operator", "Skip?"=w264) -> ("error out"=w266:errorcluster, "Login Mode Out"=w265:enum32{"Editor", "Operator"}, "Parameter Table Out"=w284:string[][], "Part Number 2"=w272:u16, "Specific Gravity Out"=w278:dbl, "Temp  Out"=w277:dbl)  [unwired: 1 out]
        "Parameter Table Out" <- w284
        "Parameter Table Out 2" <- w284
        n107 = local write "Parameter Table Out"(w284) -> ()
        n108 = case shown="\"Editor\", Default" w265 {
          tunnel: [Action."Editor Init" ("Enabled State") Action."Operator Init" ("Enabled State")] -> w285
          frame "Editor", Default {
          }
          frame "Operator" {
          }
        }
        n109 = local write "Current Configration File"(w272) -> ()
        n110 = Bundle By Name(cluster=w283, "Parameter Table Out"=w284, "Login Mode"=w265) -> (w286:T31)
        n111 = call "Enable Controls.vi"("Enabled State"=w285) -> ()  [unwired: 10 in, 1 out]
        n112 = flat-sequence {
          tunnel: w272 -> [w290]
          tunnel: w273 -> [w291]
          tunnel: [w291] -> w269
          tunnel: [w290] -> w268
          tunnel: [w289] -> w267
          tunnel: [w292] -> w271
          tunnel: w269 -> [w295]
          tunnel: w268 -> [w294]
          tunnel: w271 -> [w301]
          tunnel: T22 {"Additional Parameter Section"="ATS_Param", "Blowfish Master Password"="aztera", "Key Name"="Password", "Use Encryption"=TRUE} ("Additional Parameters Out") -> [w300]
          tunnel: w267 -> [w302]
          tunnel: w265 -> [w304]
          frame #0 {
            n113 = local read "Test Timing Mode"() -> (w289:T18)
          }
          frame #1 {
            n114 = Index Array(array=w295, index=w294) -> (element=w296:string)
            n115 = Bundle By Name(cluster=T41 {"State"=enum."By State Name", "State Name"=""} ("State Param"), "State Name"=w296) -> (w297:T41)
            n116 = call "Global VI State API.vi"("Action"=Actions."Load VI State", "State Param"=w297) -> ("Internal State Data"=w292:T29)  [unwired: 11 in, 2 out]
          }
          frame #2 {
            n117 = call "Read Additional String Parameter.vi"("Additional Parameters Out"=w300, "Internal State Data"=w301) -> ("Value"=w299:string)  [unwired: 6 in, 3 out]
            n118 = local write "Editor Password"(w299) -> ()
          }
          frame #3 {
            n119 = local write "Test Timing Mode"(w302) -> ()
            n120 = local write "Tab Control"(enum32{"Test Run", "Report ", "Graphs", "Setup"}."Test Run" ("Tab Control")) -> ()
          }
          frame #4 {
            "Login Mode Out" <- w304
          }
        }
        n121 = Bundle("Temp  Out"=w277, "Specific Gravity Out"=w278) -> (w276:T43)  [unwired: 1 in]
        n122 = call "Flow Cal_Buffer_Dbl_VIG.vi"("Constants"=w276, "SGH20"=8.32823 ("H20 Specific Gravity (h)"), "Operation"=T40."Set Ti and SGi and SGH20") -> ()  [unwired: 5 in, 4 out]
      }
      frame "Init - System" {
        # "Set Mode, then start Instrument_IO"
        n123 = Unbundle By Name(w308) -> ("Test Timing Mode"=w307:T18)
        n124 = call "Table Test Sequencer.vi"("Test Timing Mode"=w307, "Action"=StateMachineStates_TEST_TDEF."Initialize") -> ()  [unwired: 2 in, 8 out]
        n125 = Bundle By Name(cluster=w308, "DataFilePath"=path "") -> (w312:T31)
      }
      frame "Add Alarms" {
        n126 = Cluster To Array(cluster="Alarms") -> (array=w320:dbl[])
        n127 = Decimate 1D Array(w320) -> (w319:dbl[], w318:dbl[])
        n128 = Array To Cluster(array=w319) -> (cluster=w317:T44)
        n129 = Array To Cluster(array=w318) -> (cluster=w316:T44)
        n130 = call "Alarm Format Hi Lo Cluster.vi"("HI Alarm"=w317, "LO Alarm"=w316) -> ("Limits"=w323:cluster{"Lo":dbl, "Hi":dbl}[])
        n131 = call "Add Gauge Hi Lo Alarms.vi"("Action"=T26."Add Alarm Limits", "Limits"=w323) -> ()  [unwired: 9 in]
      }
      frame "----Testing-----" {
        # "This case should never run\nIt is for State Machine organization only"
      }
      frame "Set Status to Idle" {
        n132 = Bundle By Name(cluster=w333, "Test Status"=T2."Idle") -> (w332:T31)
      }
      frame "Start PID" {
        w346 = enum16{"get data", "set data", "initialize"}."set data" ("Operation")
        n133 = call "PID Active_Buffer_Bool_VIG.vi"("Operation"=enum16{"get data", "set data", "initialize"}."set data", "Boolean"=FALSE) -> ("error out"=w339:errorcluster)  [unwired: 8 in, 1 out]
        n134 = call "User BP Output_Buffer_Dbl_VIG.vi"("Operation"=w346, "Numeric"=0.0) -> ()  [unwired: 8 in, 2 out]
        n135 = call "User Current Output_Buffer_Dbl_VIG.vi"("Operation"=w346, "Numeric"=0.0) -> ()  [unwired: 8 in, 2 out]
        n136 = for {
          tunnel: string[] ["Control"] -> [w370] mode=indexing
          tunnel: [w369] -> w347
          tunnel: w339 -> [_]
          n137 = call <vilib>:"Stop Timed Structure.vi"("name"=w370) -> ("error out"=w369:errorcluster)  [unwired: 10 in]
        }
        n138 = property on="BP Regulator" class="Slide (strict)"("Value"=0.0) -> ()  [unwired: 2 in, 2 out]
        n139 = property on="Current" class="Slide (strict)"("Value"=0.0) -> ()  [unwired: 2 in, 2 out]
        n140 = flat-sequence {
          tunnel: w347 -> [w365]
          tunnel: [w365] -> w338
          frame #0 {
            n141 = call "MM_Module_Control.vi"("MM_Module_Ctrlr_Mode"=MM_Module_Control_Mode."Set", "Module Name"="Control_Loops", "MM_Module_Action In"=MM_Module_Action."Start") -> ()  [unwired: 5 in, 4 out]
          }
        }
        n142 = Tick Count (ms)() -> (millisecond timer value=w337:u32)
        n143 = while {
          tunnel: w338 -> [_]
          tunnel: w337 -> [w361]
          i -> [w354]
          stop <- w356 stop-if-true
          n144 = Wait (ms)(milliseconds to wait=u32 100) -> (millisecond timer value=w362:u32)
          n145 = Subtract(x=w362, y=w361) -> (x-y=w360:u32)
          n146 = call "PID Active_Buffer_Bool_VIG.vi"("Operation"=enum16{"get data", "set data", "initialize"}."get data") -> ("Boolean 2"=w363:bool)  [unwired: 9 in, 1 out]
          n147 = Greater?(x=w360, y=u32 60000 ("milliseconds to wait")) -> (0:w358:bool)
          n148 = Or(x=w358, y=w363) -> (x .or. y?=w355:bool)
          n149 = call "Progress.vi"("iteration"=w354, "Message"="Starting Control System...." ("String 2"), "Stop"=w355) -> ("stop"=w356:bool)  [unwired: 8 in]
        }
      }
      frame "Apply Formula" {
        n150 = for {
          tunnel: w374 -> [w386]
          tunnel: [w385] -> w373 mode=indexing
          tunnel: T42 [{"Flow Calibration Formula"=" x-0.6862*x^2+0.2588*x-0.0288", "Valid Flow Ranges"=[0.0, 0.3]}, {"Flow Calibration Formula"="x+152.23*x^6-612*x^5+1003.1*x^4 -857.22*x^3+402.56*x^2-98.486*x+9.7892", "Valid Flow Ranges"=[0.3, 1.0]}, {"Flow Calibration Formula"="x-11.943*x^4+63.453*x^3-125.22*x^2+108.76*x-35.09", "Valid Flow Ranges"=[1.0, 1.5]}, {"Flow Calibration Formula"="x+22.852*x^4-159.54*x^3+416.88*x^2-483.14*x+209.58", "Valid Flow Ranges"=[1.5, 2.0, 0.0, 0.0, 0.0, 0.0, 0.0, 0.0, 0.0, 0.0, 0.0, 0.0, 0.0, 0.0]}] -> [w381] mode=indexing
          n151 = Unbundle By Name(w381) -> ("Flow Calibration Formula"=w379:string, "Valid Flow Ranges"=w378:dbl[])
          n152 = Bundle("Flow Calibration Formula"=w379, "Specific Gravity Calibration Formula"="s+(x-t)*.0005", "Flow Conversion Formula"="Y*h*60*s") -> (w380:T45)  [unwired: 1 in]
          n153 = call "Flow Cal_Buffer_Dbl_VIG.vi"("Valid Flow Ranges"=w378, "Operation"=T40."Add New Formula", "error in"=w386, "Calibration Formulas"=w380) -> ("error out"=w385:errorcluster)  [unwired: 4 in, 3 out]
        }
        n154 = Merge Errors(w373) -> (w371:errorcluster)
      }
      frame "Start Test" {
        n155 = control-ref of="Test Table"() -> (w399:refnum<vi>)
        n156 = call "Table Color Init-Reset.vi"("Test Table"=w399) -> ()  [unwired: 11 in]
        n157 = Unbundle By Name(w390) -> ("Test Timing Mode"=w387:T18, "Number of sensors"=w389:dbl)
        n158 = control-ref of="Test Table2"() -> (w391:refnum<vi>)
        n159 = call "Table Color Init-Reset.vi"("Test Table"=w391) -> ()  [unwired: 11 in]
        n160 = Array Size(array="Test Table") -> (size(s)=w396:i32[])
        n161 = Index Array(array=w396) -> (element=w392:i32)  [unwired: 1 in]
        n162 = call "TestXYGraph_Flow_v_Current_Plot_Dbl_VIG.vi"("Plot Index/Size"=3, "Point index/size"=w392, "Operation"=T24."initialize") -> ()  [unwired: 6 in, 3 out]
        n163 = Get Date/Time String(want seconds? (F)=TRUE) -> (time string=w398:string)  [unwired: 2 in, 1 out]
        n164 = Bundle By Name(cluster=w390, "TestTable"="Test Table", "Test Status"=T2."Test Running", "Test Start Time"=w398) -> (w404:T31)
        n165 = flat-sequence {
          tunnel: w387 -> [w406]
          tunnel: w389 -> [w408]
          tunnel: "Test Table" -> [w412]
          tunnel: w387 -> [w411]
          tunnel: w387 -> [w414]
          frame #0 {
            n166 = call "Table Test Sequencer.vi"("Test Timing Mode"=w406, "Action"=StateMachineStates_TEST_TDEF."Initialize") -> ()  [unwired: 2 in, 8 out]
          }
          frame #1 {
            n167 = local read "Test Table"() -> (w410:string[][])
            n168 = call "Update Table with Sensor Data.vi"("Test Table In"=w410, "Number of Sensors"=w408) -> ("Test Table Out"=w409:string[][])  [unwired: 8 in, 5 out]
            n169 = local write "Test Table"(w409) -> ()
          }
          frame #2 {
            n170 = call "Table Test Sequencer.vi"("Test Timing Mode"=w411, "Action"=StateMachineStates_TEST_TDEF."Start", "Test Table"=w412) -> ()  [unwired: 1 in, 8 out]
          }
          frame #3 {
            n171 = case shown="\"Manual\", Default" w414 {
              selector: w414 -> [w416 _]
              tunnel: [Action."Manual Test Start" ("Enabled State") Action."Timed Test Start" ("Enabled State")] -> w415
              frame "Manual", Default {
                n172 = call "Table Test Sequencer.vi"("Test Timing Mode"=w416, "Action"=StateMachineStates_TEST_TDEF."Pause") -> ()  [unwired: 2 in, 8 out]
              }
              frame "Automatic" {
              }
            }
            n173 = call "Enable Controls.vi"("Enabled State"=w415) -> ()  [unwired: 10 in, 1 out]
          }
        }
        n174 = call "concatinate 2 strings with linefeed.vi"("String 2"="Run Test" ("element"), "String 1"=w402) -> ("Concatinated OUT"=w401:string)  [unwired: 6 in]
      }
      frame "Pause Test" {
        n175 = Bundle By Name(cluster=w425, "Test Status"=T2."Test Paused") -> (w424:T31)
        n176 = call "Table Test Sequencer.vi"("Action"=StateMachineStates_TEST_TDEF."Pause") -> ()  [unwired: 3 in, 8 out]
      }
      frame "Resume Test" {
        w429 = T2."Test Running"  # Test Status
        n177 = Bundle By Name(cluster=w432, "Test Status"=w429) -> (w431:T31)
        n178 = call "Table Test Sequencer.vi"("Action"=StateMachineStates_TEST_TDEF."Resume") -> ()  [unwired: 3 in, 8 out]
      }
      frame "Stop Test" {
        n179 = Unbundle By Name(w436) -> ("Login Mode"=w435:enum32{"Editor", "Operator"})
        n180 = case shown="\"Operator\"" w435 {
          tunnel: [Action."Editor Init" ("Enabled State") Action."Operator Init" ("Enabled State")] -> w437
          frame "Editor", Default {
          }
          frame "Operator" {
          }
        }
        n181 = call "Enable Controls.vi"("Enabled State"=w437) -> ()  [unwired: 10 in, 1 out]
        n182 = Get Date/Time String(want seconds? (F)=TRUE) -> (time string=w439:string)  [unwired: 2 in, 1 out]
        n183 = Bundle By Name(cluster=w436, "Test Status"=T2."Test Completed", "Test Stop Time"=w439) -> (w442:T31)
        n184 = flat-sequence {
          frame #0 {
            n185 = control-ref of="Test Table"() -> (w448:refnum<vi>)
            n186 = control-ref of="Test Table2"() -> (w447:refnum<vi>)
            n187 = call "Table Test Sequencer.vi"("Action"=StateMachineStates_TEST_TDEF."Get Step") -> ("Current Step ID"=w446:i32)  [unwired: 3 in, 7 out]
            n188 = call "Table Color Clear Select.vi"("Current Step ID"=w446, "Test Table"=w448) -> ()  [unwired: 10 in]
            n189 = call "Table Color Clear Select.vi"("Current Step ID"=w446, "Test Table"=w447) -> ()  [unwired: 10 in]
          }
          frame #1 {
            n190 = control-ref of="Test Table"() -> (w450:refnum<vi>)
            n191 = call "Table Color Init-Reset.vi"("Test Table"=w450) -> ()  [unwired: 11 in]
          }
        }
      }
      frame "Run Test" {
        # "VIG for Data\n(Flow-I) plot"
        n192 = Unbundle By Name(w453) -> ("Test Timing Mode"=w451:T18, "DataFilePath"=w473:path, "Test Status"=w461:T2, "Number of sensors"=w452:dbl)
        n193 = local read "Test Table"() -> (w465:string[][])
        n194 = control-ref of="Test Table"() -> (w469:refnum<vi>)
        n195 = call "Table Test Sequencer.vi"("Test Timing Mode"=w451, "Action"=StateMachineStates_TEST_TDEF."Run Position") -> ("Test Running"=w462:bool, "Current Step ID"=w454:i32)  [unwired: 2 in, 6 out]
        n196 = call "Table Color Update.vi"("Value"=w465, "Current Step ID"=w454, "Test Table"=w469) -> ("Current Setpoint (mA)"=w455:dbl, "Min and Max Flow Alarm"=w458:cluster{"Min":dbl, "Max":dbl})  [unwired: 7 in]
        n197 = Unbundle By Name(w458) -> ("Min"=w457:dbl, "Max"=w456:dbl)
        n198 = property on="Flow 2" class="DigNum (strict)"("Value"=w457) -> ()  [unwired: 2 in, 2 out]
        n199 = property on="Flow" class="DigNum (strict)"("Value"=w456) -> ()  [unwired: 2 in, 2 out]
        n200 = call "Update Table with Sensor Data.vi"("Test Table In"=w465, "Number of Sensors"=w452) -> ("CountDown Clock"=→"CountDown Pie":picture, "Test Table Out"=w464:string[][], "Test Timing Mode"=w459:enum16{"Manual", "Timed"}, "CountDown Text"=→"CountDown Text":string)  [unwired: 8 in, 2 out]
        "Test Table2" <- w464
        n201 = case shown="\"Test Running\"" w461 {
          selector: w461 -> [w480 _]
          tunnel: w462 -> [_ w487]
          tunnel: [w480 w486] -> w460
          tunnel: w459 -> [_ w483]
          tunnel: w455 -> [_ w482]
          tunnel: w453 -> [_ w485]
          frame "Idle", Default {
          }
          frame "Test Running" {
            n202 = local read "Current Manual Control"() -> (w481:bool)
            n203 = Select(t=T2."Test Running" ("Test Status"), s=w487, f=T2."Test Completed" ("Test Status")) -> (s? t:f=w486:T2)
            n204 = case shown="False" w481 {
              tunnel: w482 -> [w491 _]
              frame False {
                n205 = call "User Current Output_Buffer_Dbl_VIG.vi"("Operation"=enum16{"get data", "set data", "initialize"}."set data", "Numeric"=w491) -> ()  [unwired: 8 in, 2 out]
              }
              frame True {
              }
            }
            n206 = Unbundle By Name(w485) -> ("Test Timing Mode"=w484:T18)
            n207 = case shown="\"Semi-Automatic\"" w484 {
              selector: w484 -> [_ _ w492]
              tunnel: w483 -> [_ _ w495]
              frame "Manual", Default {
              }
              frame "Automatic" {
              }
              frame "Semi-Automatic" {
                n208 = case shown="\"Manual\", Default" w495 {
                  tunnel: [StateMachineStates_TEST_TDEF."Pause" ("Action") StateMachineStates_TEST_TDEF."Resume" ("Action")] -> w494
                  tunnel: [Action."Manual Test Start" ("Enabled State") Action."Timed Test Start" ("Enabled State")] -> w493
                  frame "Manual", Default {
                    w497 = Timer_Actions_ENUM_TEST_TDef."Set Time"  # Timer Action
                    n209 = call "Timer With Pause.vi"("Timer Action"=w497, "Target Time"=0.0) -> ()  [unwired: 6 in, 4 out]
                  }
                  frame "Timed" {
                  }
                }
                n210 = call "Enable Controls.vi"("Enabled State"=w493) -> ()  [unwired: 10 in, 1 out]
                n211 = call "Table Test Sequencer.vi"("Test Timing Mode"=w492, "Action"=w494) -> ()  [unwired: 2 in, 8 out]
              }
            }
          }
        }
        n212 = Bundle By Name(cluster=w453, "queue data.Variant Data"=variant, "Calibrate"=FALSE, "Test Status"=w460) -> (w477:T31)
        n213 = local write "Test Table"(w464) -> ()
        n214 = flat-sequence {
          tunnel: w454 -> [w503]
          tunnel: w464 -> [w502]
          frame #0 {
            n215 = control-ref of="Test Table2"() -> (w504:refnum<vi>)
            n216 = call "Table Color Update.vi"("Value"=w502, "Current Step ID"=w503, "Test Table"=w504) -> ()  [unwired: 7 in, 2 out]
          }
        }
        n217 = call "Tag_Buffer_Dbl_Input_VIG.vi"("Operation"=enum16{"get data", "set data", "initialize"}."get data") -> ("tag_data_out"=w470:dbl[])  [unwired: 9 in, 1 out]
        n218 = Number To Fractional String(number=w470) -> (F-format string=w471:string[])  [unwired: 3 in]
        n219 = Path To String(path=w473) -> (string=w474:string)
        n220 = case shown="\"<Not A Path>\"" w474 {
          tunnel: w472 -> [w505 w510]
          tunnel: [w505 w509] -> _
          tunnel: w471 -> [_ w506]
          tunnel: w473 -> [_ w508]
          frame "<Not A Path>" {
          }
          frame "", Default {
            n221 = call "WRIS Write To Spreadsheet File (string) with Error Clusters.vi"("file path (dialog if empty)"=w508, "1D data"=w506, "error in"=w510, "append to file? (new file:F)"=TRUE ("transpose? (no:F)")) -> ("error out"=w509:errorcluster)  [unwired: 10 in, 1 out]
          }
        }
      }
      frame "----- Processing -----" {
        # "This case should never run\nIt is for State Machine organization only"
      }
      frame "Send to Excel" {
        n222 = Unbundle By Name(w518) -> ("Parameter Table Out"=w523:string[][], "Test Start Time"=w521:string, "Test Stop Time"=w520:string)
        n223 = local read "Test Table"() -> (w522:string[][])
        n224 = call "Generate ATS Excel Report.vi"("Test_Start_Time"=w521, "Additional Report Values"="Additional Report Values", "Test_End_Time"=w520, "start path"=path "c:/Torque Motor Reports", "template (empty)"=path "C:/Torque Motor Report Templates/3882506-6 Template.xls", "Test Table"=w522, "Parameter Table Out"=w523) -> ()  [unwired: 5 in]
      }
      frame "Wait" {
        n225 = Decimal String To Number(string=w529, default (0L)=1000 ("default (0 I32)")) -> (number=w527:i32)  [unwired: 1 in, 1 out]
        n226 = Wait (ms)(milliseconds to wait=w527) -> ()  [unwired: 1 out]
      }
    }
    n227 = Unbundle By Name(w84) -> ("Test Status"=→"Test Status":T2)
  }
  n228 = while "User Events" {
    tunnel: w2 -> [w534]
    tunnel: w6 -> [w533]
    tunnel: [TRUE] -> _
    stop <- w535 stop-if-true
    n229 = event shown="[22] \"Control Devices\": Value Change" {
      selector: _ -> [_ _ _ _ _ _ _ _ _ _ _ _ _ _ _ _ _ _ _ _ _ _ _ _]
      dyn-events: _ -> [_ _ _ _ _ _ _ _ _ _ _ _ _ _ _ _ _ _ _ _ _ _ _ _]
      timeout: w533 -> [_ _ _ _ _ _ _ _ _ _ _ _ _ _ _ _ _ _ _ _ _ _ _ _]
      tunnel: [_ _ _ _ "Exit" TRUE ("Exit") _ _ _ _ _ _ _ _ _ _ _ _ _ _ _ _ _ _] -> w535
      tunnel: w534 -> [_ w584 _ w590 w595 w600 w603 w607 w611 _ _ w656 _ _ _ w735 _ _ w749 w751 w754 w757 _ w765]
      event Timeout {
        w553 = enum16{"get data", "set data", "initialize"}."get data" ("Operation")
        n230 = event-data() -> ()  [unwired: 1 in, 2 out]
        n231 = control-ref of="Test Table2"() -> (w566:refnum<vi>)
        n232 = property on="Test Table" class="Tbl (strict)"() -> ("EditPos"=w571:T47)  [unwired: 2 in, 2 out]
        n233 = local read "BP Regulator Manual Control"() -> (w551:bool)
        n234 = call "Update Row Headers.vi"("Test Table"=w566) -> ()
        n235 = call "PID SP_Buffer_Dbl_VIG.vi"("Operation"=enum16{"get data", "set data", "initialize"}."set data", "Numeric"="Setpoint (psid)") -> ()  [unwired: 8 in, 2 out]
        n236 = local read "Current Manual Control"() -> (w550:bool)
        n237 = control-ref of="Test Table"() -> (w569:refnum<vi>)
        n238 = Unbundle(w571) -> ("Row"=w559:i32, "Column"=→"EditCol":i32)
        "EditLine" <- w559
        n239 = call "Update Row Headers.vi"("Test Table"=w569) -> ()
        n240 = call "PID Tolerance_Buffer_Dbl_VIG.vi"("Operation"=enum16{"get data", "set data", "initialize"}."set data", "Numeric"="Tolerance (psid)") -> ()  [unwired: 8 in, 2 out]
        n241 = case shown="False" w551 {
          frame False {
            n242 = call "PID Output_Buffer_Dbl_VIG.vi"("Operation"=T25."get data") -> ("Numeric"=w574:dbl)  [unwired: 9 in, 1 out]
            n243 = Divide(x=w574, y=300.0) -> (x/y=w573:dbl)
            n244 = property on="BP Regulator" class="Slide (strict)"("Value"=w573) -> ()  [unwired: 2 in, 2 out]
          }
          frame True {
          }
        }
        n245 = case shown="False" w550 {
          frame False {
            n246 = call "User Current Output_Buffer_Dbl_VIG.vi"("Operation"=enum16{"get data", "set data", "initialize"}."get data") -> ("Numeric"=w576:dbl)  [unwired: 9 in, 1 out]
            n247 = property on="Current" class="Slide (strict)"("Value"=w576) -> ()  [unwired: 2 in, 2 out]
          }
          frame True {
          }
        }
        n248 = case shown="-2" w559 {
          tunnel: w559 -> [_ w578]
          frame -2 {
          }
          frame 1, Default {
            n249 = Bundle("Row"=w578, 0) -> (w580:cluster{"Row":i32, i32})  [unwired: 1 in]
            n250 = Bundle(1, 6) -> (w579:cluster{i32, i32})  [unwired: 1 in]
            n251 = property on="Test Table" class="Tbl (strict)"("Selection Start"=w580, "Selection Size"=w579) -> ()  [unwired: 2 in, 2 out]
          }
        }
        n252 = call "PID In Range_Buffer_Bool_VIG.vi"("Operation"=enum16{"get data", "set data", "initialize"}."get data") -> ("Current in tol?"=→"Current within Tolerance":bool, "Boolean 2"=→"Diff. Press within Tolerance":bool)  [unwired: 8 in, 1 out]
        n253 = call "Add Gauge Hi Lo Alarms.vi"("Action"=T26."Check for Alarm") -> ()  [unwired: 10 in]
        n254 = call "Tag_Buffer_Dbl_Input_VIG.vi"("Operation"=enum16{"get data", "set data", "initialize"}."get data") -> ("tag_data_out"=w564:dbl[])  [unwired: 9 in, 1 out]
        n255 = call "Agilent_Buffer_Dbl_VIG.vi"("Operation"=w553) -> ("Numeric"=→"Actual Current":dbl)  [unwired: 9 in, 1 out]
        n256 = call "Table Test Sequencer.vi"("Action"=StateMachineStates_TEST_TDEF."Get Step") -> ("Current Step ID"=w561:i32)  [unwired: 3 in, 7 out]
        n257 = call "Format Data Buffer to Cluster.vi"("tag_data_out"=w564) -> ("Analog Sensors"=→"Analog Sensors":T3)  [unwired: 1 out]
        n258 = call "TestXYGraph_Flow_v_Current_Plot_Dbl_VIG.vi"("Point index/size"=w561, "Operation"=T24."get data") -> ("XY Graph"=→"Flow-Current XY Graph":cluster{cluster{"X":dbl, "Y":dbl}[]}[])  [unwired: 7 in, 2 out]
        n259 = call "Agilent_Volt_Buffer_Dbl_VIG.vi"("Operation"=w553) -> ("Numeric"=→"Actual  Voltage":dbl)  [unwired: 9 in, 1 out]
        n260 = call "Tag_InstrIO_Error_VIG.vi"("Operation"=enum16{"get data", "set data", "initialize"}."get data") -> ("Error Status"=w546:bool[], "tag_data_out"=w557:errorcluster[])  [unwired: 9 in]
        n261 = Index Array(array=w557) -> (element #1=→"USB 6211":errorcluster, element #2=→"USB Agilent":errorcluster, element #3=→"USB TC 01":errorcluster, element #4=→"FEM-03":errorcluster)  [unwired: 4 in]
        n262 = Index Array(array=w546) -> (element #1=→"DAQ":bool, element #2=→"Agilent":bool, element #3=→"Thermocouple":bool, element #4=→"Flow Meter":bool)  [unwired: 4 in]
      }
      event Key Down; "Alarms": Value Change {
        n263 = event-data() -> ()  [unwired: 1 in, 3 out]
        n264 = call "Queue Command Bundle.vi"("Command"="Add Alarms" ("element")) -> ("main window queue datatype"=w585:T32)  [unwired: 10 in]
        n265 = Enqueue Element(queue=w584, element=w585) -> ()  [unwired: 2 in, 3 out]
      }
      event "Test Table": Key Down? {
        n266 = event-data() -> ()  [unwired: 1 in, 9 out]
        n267 = local read "Login Mode Out"() -> (w589:enum32{"Editor", "Operator"})
        n268 = Equal?(x=w589, y=enum32{"Editor", "Operator"}."Operator") -> (x = y?=w587:bool)
        n269 = event-data("Discard?"=w587) -> ()  [unwired: 6 in, 1 out]
      }
      event "Enable": Value Change {
        n270 = event-data() -> ()  [unwired: 1 in, 5 out]
        n271 = call "Queue Command Bundle.vi"("Command"="Alarm Enable?" ("element")) -> ("main window queue datatype"=w591:T32)  [unwired: 10 in]
        n272 = Enqueue Element(queue=w590, element=w591) -> ()  [unwired: 2 in, 3 out]
      }
      event "Exit": Value Change; Application Instance Close {
        n273 = event-data() -> ()  [unwired: 1 in, 3 out]
        n274 = call "Queue Command Bundle.vi"("Command"="Exit" ("element")) -> ("main window queue datatype"=w593:T32)  [unwired: 10 in]
        n275 = Enqueue Element(queue=w595, element=w593) -> ()  [unwired: 2 in, 3 out]
      }
      event Panel Close {
        n276 = event-data() -> ()  [unwired: 1 in, 4 out]
        n277 = call "Queue Command Bundle.vi"("Command"="Exit" ("element")) -> ("main window queue datatype"=w598:T32)  [unwired: 10 in]
        n278 = Enqueue Element(queue=w600, element=w598) -> ()  [unwired: 2 in, 3 out]
      }
      event "StartTest": Value Change {
        n279 = event-data() -> ()  [unwired: 1 in, 5 out]
        n280 = call "Queue Command Bundle.vi"("Command"="Get Initial Constants\nReset IO\nStart PID\nSet Manual Controls\nChange Timing Mode\nStart Test" ("element")) -> ("main window queue datatype"=w601:T32)  [unwired: 10 in]
        n281 = Enqueue Element(queue=w603, element=w601) -> ()  [unwired: 2 in, 3 out]
      }
      event "StopTest": Value Change {
        n282 = event-data() -> ()  [unwired: 1 in, 5 out]
        n283 = call "Queue Command Bundle.vi"("Command"="Stop Test" ("element")) -> ("main window queue datatype"=w605:T32)  [unwired: 10 in]
        n284 = call "Table Test Sequencer.vi"("Action"=StateMachineStates_TEST_TDEF."Initialize") -> ()  [unwired: 3 in, 8 out]
        n285 = Enqueue Element(queue=w607, element=w605) -> ()  [unwired: 2 in, 3 out]
      }
      event "PauseTest": Value Change {
        n286 = event-data() -> ()  [unwired: 1 in, 6 out]
        n287 = Select(t="Pause Test" ("element"), s="PauseTest", f="Resume Test" ("element")) -> (s? t:f=w608:string)
        n288 = call "Queue Command Bundle.vi"("Command"=w608) -> ("main window queue datatype"=w612:T32)  [unwired: 10 in]
        n289 = Enqueue Element(queue=w611, element=w612) -> ()  [unwired: 2 in, 3 out]
      }
      event Value Change {
        n290 = event-data() -> ("CtlRef"=w616:refnum<vi>)  [unwired: 1 in, 5 out]
        n291 = property class="Bool"(reference=w616) -> ("Label.Text"=w615:string)  [unwired: 1 in, 2 out]
        n292 = case shown="\"New\", Default" w615 {
          tunnel: "FileGroup_1" -> [_ _ _]
          frame "New", Default {
            (unwired) ""
            # "Need to prompt for saving current table\nif changed."
            n293 = Initialize Array("", 1, 6) -> (w617:string[][])
            n294 = global write "FFT_DAS-Editing Variables_GBL.vi" "TestTable Changed"(FALSE) -> ()
            n295 = local write "Test Table"(w617) -> ()
          }
          frame "Open" {
            (unwired) ""
            # "Need to prompt for saving current table\nif changed."
            n296 = call <userlib>:"Current VIs Parent Directory__ogtk.vi"("Relative path (.)"=path "Config_Files") -> ("Parent Directory (+ Relative)"=w628:path)  [unwired: 4 in]
            n297 = call "File Dialog3"("start path"=w628, "prompt"="Enter File Name to Open", "default name"="Test Steps.txt") -> ("selected path"=w625:path)  [unwired: 9 in, 3 out]
            n298 = call-poly <vilib>:"Read From Spreadsheet File.vi"("format (%s)"="%s", "file path (dialog if empty)"=w625) -> ("all rows"=w623:string[][])  [unwired: 5 in, 4 out]
            n299 = local write "Test Table"(w623) -> ()
            n300 = global write "FFT_DAS-Editing Variables_GBL.vi" "TestTable Changed"(FALSE) -> ()
          }
          frame "Save" {
            n301 = call <userlib>:"Current VIs Parent Directory__ogtk.vi"("Relative path (.)"=path "Config_Files") -> ("Parent Directory (+ Relative)"=w634:path)  [unwired: 4 in]
            n302 = call "File Dialog2"("start path"=w634, "prompt"="Enter File Name to Save As", "default name"="Test Steps.txt") -> ("selected path"=w631:path, "cancelled"=w632:bool)  [unwired: 9 in, 2 out]
            n303 = case shown="False" w632 {
              tunnel: w631 -> [w638 _]
              frame False {
                n304 = local read "Test Table"() -> (w637:string[][])
                n305 = call-poly <vilib>:"Write To Spreadsheet File.vi"("format (%s)"="%s", "2D data"=w637, "file path (dialog if empty)"=w638) -> ()  [unwired: 5 in, 1 out]
              }
              frame True {
              }
            }
          }
        }
      }
      event Value Change {
        n306 = event-data() -> ()  [unwired: 1 in, 6 out]
        n307 = property on="Current Configration File" class="Ring (strict)"() -> ("Strings []"=w645:string[])  [unwired: 2 in, 2 out]
        n308 = local read "Current Configration File"() -> (w644:u16)
        n309 = Index Array(array=w645, index=w644) -> (element=w641:string)
        n310 = Concatenate Strings("Do you want to delete configuration for SN  " ("message"), w641, "?" ("string")) -> (w643:string)
        n311 = Two Button Dialog(message=w643, 2:"Delete" ("T button name (\"OK\")")) -> (T button?=w640:bool)  [unwired: 1 in]
        n312 = case shown="True" w640 {
          tunnel: w641 -> [_ w652]
          tunnel: w644 -> [_ w651]
          frame False {
          }
          frame True {
            n313 = Bundle By Name(cluster=T41 {"State"=enum."By State Name", "State Name"=""} ("State Param"), "State Name"=w652) -> (w653:T41)
            n314 = Decrement(x=w651) -> (x-1=w650:u16)
            n315 = local write "Current Configration File"(w650) -> ()
            n316 = call "Global VI State API.vi"("Action"=Actions."Delete State", "State Param"=w653) -> ("Error"=w647:errorcluster)  [unwired: 11 in, 2 out]
            n317 = call "Global VI State API.vi"("Action"=Actions."Get All VI State Names", "Error In"=w647) -> ("VI States"=w648:string[])  [unwired: 11 in, 2 out]
            n318 = property on="Current Configration File" class="Ring (strict)"("Strings []"=w648) -> ()  [unwired: 2 in, 2 out]
          }
        }
      }
      event Value Change {
        n319 = event-data() -> ("CtlRef"=w657:refnum<vi>)  [unwired: 1 in, 5 out]
        n320 = property class="Bool"(reference=w657) -> ("Label.Text"=w658:string)  [unwired: 1 in, 2 out]
        n321 = case shown="\"New\", Default" w658 {
          tunnel: "Current Configration File" -> [_ w671 w680]
          tunnel: w656 -> [_ w670 w679]
          frame "New", Default {
            n322 = call "Save Configuration File For Part Number"() -> ("Part Number"=w661:string, "Save"=w660:bool)  [unwired: 17 in, 1 out]
            n323 = case shown="True" w660 {
              tunnel: w661 -> [_ w666]
              tunnel: [Actions."Get All VI State Names" ("Action") Actions."Get All VI State Names" ("Action")] -> w662
              frame False {
              }
              frame True {
                n324 = Bundle By Name(cluster=T41 {"State"=enum."By State Name", "State Name"=""} ("State Param"), "State Name"=w666) -> (w667:T41)
                n325 = call "Global VI State API.vi"("Action"=Actions."Save VI State", "State Param"=w667) -> ()  [unwired: 11 in, 3 out]
              }
            }
            n326 = call "Global VI State API.vi"("Action"=w662) -> ("VI States"=w663:string[])  [unwired: 12 in, 2 out]
            n327 = property on="Current Configration File" class="Ring (strict)"("Strings []"=w663) -> ()  [unwired: 2 in, 2 out]
          }
          frame "Open" {
            n328 = property on="Current Configration File" class="Ring (strict)"() -> ("Strings []"=w672:string[])  [unwired: 2 in, 2 out]
            n329 = call "Queue Command Bundle.vi"("Command"="Add Alarms\nAlarm Enable?\nApply Formula\nReset IO\nStart PID" ("element")) -> ("main window queue datatype"=w678:T32)  [unwired: 10 in]
            n330 = Enqueue Element(queue=w670, element=w678) -> ()  [unwired: 2 in, 3 out]
            n331 = Index Array(array=w672, index=w671) -> (element=w676:string)
            n332 = Bundle By Name(cluster=T41 {"State"=enum."By State Name", "State Name"=""} ("State Param"), "State Name"=w676) -> (w675:T41)
            n333 = call "Global VI State API.vi"("Action"=Actions."Load VI State", "State Param"=w675) -> ()  [unwired: 11 in, 3 out]
          }
          frame "Save" {
            n334 = property on="Current Configration File" class="Ring (strict)"() -> ("Strings []"=w681:string[])  [unwired: 2 in, 2 out]
            n335 = call "Queue Command Bundle.vi"("Command"="Add Alarms\nAlarm Enable?\nApply Formula\nReset IO\nStart PID" ("element")) -> ("main window queue datatype"=w687:T32)  [unwired: 10 in]
            n336 = Enqueue Element(queue=w679, element=w687) -> ()  [unwired: 2 in, 3 out]
            n337 = Index Array(array=w681, index=w680) -> (element=w685:string)
            n338 = Bundle By Name(cluster=T41 {"State"=enum."By State Name", "State Name"=""} ("State Param"), "State Name"=w685) -> (w684:T41)
            n339 = call "Global VI State API.vi"("Action"=Actions."Save VI State", "State Param"=w684) -> ()  [unwired: 11 in, 3 out]
          }
        }
      }
      event Value Change {
        (unwired) enum16{"Cut", "Copy", "Paste"}."Paste"
        n340 = event-data() -> ("CtlRef"=w691:refnum<vi>)  [unwired: 1 in, 5 out]
        n341 = property class="Bool"(reference=w691) -> ("Label.Text"=w690:string)  [unwired: 1 in, 2 out]
        n342 = case shown="\"Cut\", \"Delete\", Default" w690 {
          tunnel: "EditGroup_1" -> [_ _ _]
          tunnel: "Delete" -> [w692 _ _]
          frame "Cut", "Delete", Default {
            n343 = local read "Test Table"() -> (w695:string[][])
            n344 = property on="Test Table" class="Tbl (strict)"() -> ("Selection Start"=w697:T47, "Selection Size"=w696:T47)  [unwired: 2 in, 2 out]
            n345 = call "Table Function - Cut to Ext-Clipboard.vi"("Selection Size"=w696, "Selection Start"=w697, "Text Table"=w695) -> ("Cut Section to Clipboard"=w693:string[][], "Table minus Cut Section"=w694:string[][])  [unwired: 6 in, 1 out]
            n346 = global write "FFT_DAS-Editing Variables_GBL.vi" "TestTable Changed"(TRUE) -> ()
            n347 = case shown="False" w692 {
              tunnel: w693 -> [w699 _]
              frame False {
                n348 = global write "FFT_DAS-Editing Variables_GBL.vi" "T-Tbl Clpbd"(w699) -> ()
              }
              frame True {
              }
            }
            n349 = local write "Test Table"(w694) -> ()
          }
          frame "Copy" {
            n350 = local read "Test Table"() -> (w702:string[][])
            n351 = property on="Test Table" class="Tbl (strict)"() -> ("Selection Start"=w704:T47, "Selection Size"=w703:T47)  [unwired: 2 in, 2 out]
            n352 = call "Table Function - Copy to Ext-Clipboard.vi"("Selection Size"=w703, "Selection Start"=w704, "Text Table In"=w702) -> ("Cut Section to Clipboard"=w700:string[][], "Text Table Out"=w701:string[][])  [unwired: 6 in, 1 out]
            n353 = global write "FFT_DAS-Editing Variables_GBL.vi" "TestTable Changed"(TRUE) -> ()
            n354 = global write "FFT_DAS-Editing Variables_GBL.vi" "T-Tbl Clpbd"(w700) -> ()
            n355 = local write "Test Table"(w701) -> ()
          }
          frame "Paste" {
            n356 = local read "Test Table"() -> (w708:string[][])
            n357 = property on="Test Table" class="Tbl (strict)"() -> ("Selection Start"=w710:T47, "Selection Size"=w709:T47)  [unwired: 2 in, 2 out]
            n358 = global read "FFT_DAS-Editing Variables_GBL.vi" "T-Tbl Clpbd"() -> (w706:string[][])
            n359 = call "Table Function - Paste from Ext-Clipboard.vi"("Cut Section from Clipboard"=w706, "Selection Size"=w709, "Selection Start"=w710, "Text Table In"=w708) -> ("Text Table Out"=w707:string[][])  [unwired: 6 in, 1 out]
            n360 = global write "FFT_DAS-Editing Variables_GBL.vi" "TestTable Changed"(TRUE) -> ()
            n361 = local write "Test Table"(w707) -> ()
          }
        }
      }
      event Value Change {
        n362 = event-data() -> ("CtlRef"=w715:refnum<vi>)  [unwired: 1 in, 5 out]
        n363 = property on="Test Table" class="Tbl (strict)"() -> ("EditPos"=w713:T47)  [unwired: 2 in, 2 out]
        n364 = property class="Bool"(reference=w715) -> ("Label.Text"=w714:string)  [unwired: 1 in, 2 out]
        n365 = Unbundle(w713) -> ("Row"=w712:i32)  [unwired: 1 out]
        n366 = case shown="\"Block Start\", Default" w714 {
          tunnel: w712 -> [w716 w719]
          frame "Block Start", Default {
            n367 = global write "FFT_DAS-Editing Variables_GBL.vi" "Block Start"(w716) -> ()
          }
          frame "Block End" {
            n368 = global read "FFT_DAS-Editing Variables_GBL.vi" "Block Start"() -> (w718:i32)
            n369 = global write "FFT_DAS-Editing Variables_GBL.vi" "Block End"(w719) -> ()
            n370 = Equal?(x=w719, y=w718) -> (x = y?=w717:bool)
            n371 = case shown="False" w717 {
              tunnel: w719 -> [w723 _]
              tunnel: w718 -> [w722 _]
              frame False {
                n372 = Subtract(x=w723, y=w722) -> (x-y=w726:i32)
                n373 = Increment(x=w726) -> (x+1=w727:i32)
                n374 = Bundle("Block Start"=w722, 0) -> (w721:cluster{"Block Start":i32, i32})  [unwired: 1 in]
                n375 = Bundle(w727, 6) -> (w720:cluster{i32, i32})  [unwired: 1 in]
                n376 = global write "FFT_DAS-Editing Variables_GBL.vi" "Block Select"(TRUE) -> ()
                n377 = property on="Test Table" class="Tbl (strict)"("Selection Start"=w721, "Selection Size"=w720) -> ()  [unwired: 2 in, 2 out]
              }
              frame True {
              }
            }
          }
        }
      }
      event "MacroGroup.MacroName": Value Change {
        n378 = event-data() -> ("CtlRef"=w731:refnum<vi>)  [unwired: 1 in, 5 out]
        n379 = property class="Ctl"(reference=w731) -> ("Label.Text"=w729:string)  [unwired: 1 in, 2 out]
        n380 = case shown="\"MacroName\"" w729 {
          tunnel: "MacroGroup" -> [_ _ _ _]
          frame "MacroPlay", Default {
          }
          frame "MacroPause" {
          }
          frame "MacroStop" {
          }
          frame "MacroName" {
          }
        }
      }
      event Value Change {
        n381 = event-data() -> ()  [unwired: 1 in, 3 out]
        n382 = To Variant(anything="Test Timing Mode") -> (Variant=w733:variant)
        n383 = call "Queue Command Bundle.vi"("Variant Data"=w733, "Command"="Change Timing Mode" ("element")) -> ("main window queue datatype"=w736:T32)  [unwired: 9 in]
        n384 = Enqueue Element(queue=w735, element=w736) -> ()  [unwired: 2 in, 3 out]
      }
      event "Go to Next Step": Value Change {
        n385 = event-data() -> ()  [unwired: 1 in, 3 out]
        n386 = local read "Test Timing Mode"() -> (w737:T18)
        n387 = disable-structure shown="Disabled" {
          frame Disabled {
            n388 = call "Timer With Pause.vi"("Timer Action"=Timer_Actions_ENUM_TEST_TDef."Set Time", "Target Time"=0.0) -> ()  [unwired: 6 in, 4 out]
          }
          frame Enabled {
          }
        }
        n389 = call "Table Test Sequencer.vi"("Test Timing Mode"=w737, "Action"=StateMachineStates_TEST_TDEF."Force Next Step") -> ()  [unwired: 2 in, 8 out]
      }
      event "Save Password": Value Change {
        n390 = event-data() -> ()  [unwired: 1 in, 3 out]
        n391 = call "Global VI State API.vi"("Action"=Actions."Get All VI State Names") -> ("Internal State Data"=w746:T29, "Error"=w743:errorcluster)  [unwired: 12 in, 1 out]
        n392 = call "Write Additional String Parameter.vi"("error in (no error)"=w743, "value"="Editor Password", "Additional Parameters Out"=T22 {"Additional Parameter Section"="ATS_Param", "Blowfish Master Password"="aztera", "Key Name"="Password", "Use Encryption"=TRUE}, "Internal State Data"=w746) -> ("error out"=w741:errorcluster)  [unwired: 5 in, 2 out]
        n393 = call "Global VI State API.vi"("Action"=Actions."Write Data to File", "Error In"=w741) -> ()  [unwired: 11 in, 3 out]
      }
      event "Current Manual Control", "BP Regulator Manual Control": Value Change {
        n394 = event-data() -> ()  [unwired: 1 in, 3 out]
        n395 = call "Queue Command Bundle.vi"("Command"="Set Manual Controls" ("element")) -> ("main window queue datatype"=w750:T32)  [unwired: 10 in]
        n396 = Enqueue Element(queue=w749, element=w750) -> ()  [unwired: 2 in, 3 out]
      }
      event "Simulate Hardware", "Agilent Resource Name", "FEM-03 Port", "System Refresh Button", "reset", "Rest All IO": Value Change {
        n397 = event-data() -> ()  [unwired: 1 in, 3 out]
        n398 = call "Queue Command Bundle.vi"("Command"="Reset IO" ("element")) -> ("main window queue datatype"=w752:T32)  [unwired: 10 in]
        n399 = Enqueue Element(queue=w751, element=w752) -> ()  [unwired: 2 in, 3 out]
      }
      event "Send PID": Value Change {
        n400 = event-data() -> ()  [unwired: 1 in, 3 out]
        n401 = call "Queue Command Bundle.vi"("Command"="Start PID" ("element")) -> ("main window queue datatype"=w755:T32)  [unwired: 10 in]
        n402 = Enqueue Element(queue=w754, element=w755) -> ()  [unwired: 2 in, 3 out]
      }
      event "Stability Dwell Time (sec)": Value Change {
        n403 = event-data() -> ()  [unwired: 1 in, 3 out]
        n404 = call "Queue Command Bundle.vi"("Command"="Set Stability Time" ("element")) -> ("main window queue datatype"=w758:T32)  [unwired: 10 in]
        n405 = Enqueue Element(queue=w757, element=w758) -> ()  [unwired: 2 in, 3 out]
      }
      event "Control Devices": Value Change {
        w762 = enum16{"get data", "set data", "initialize"}."set data" ("Operation")
        n406 = event-data() -> ()  [unwired: 1 in, 3 out]
        n407 = Cluster To Array(cluster="Control Devices") -> (array=w763:dbl[])
        n408 = Index Array(array=w763) -> (element #1=w761:dbl, element #2=w760:dbl)  [unwired: 2 in]
        n409 = call "User Current Output_Buffer_Dbl_VIG.vi"("Operation"=w762, "Numeric"=w761) -> ()  [unwired: 8 in, 2 out]
        n410 = call "User BP Output_Buffer_Dbl_VIG.vi"("Operation"=w762, "Numeric"=w760) -> ()  [unwired: 8 in, 2 out]
      }
      event "Send to Excel": Value Change {
        n411 = event-data() -> ()  [unwired: 1 in, 6 out]
        n412 = call "Queue Command Bundle.vi"("Command"="Send to Excel" ("element")) -> ("main window queue datatype"=w766:T32)  [unwired: 10 in]
        n413 = Enqueue Element(queue=w765, element=w766) -> ()  [unwired: 2 in, 3 out]
      }
    }
  }
  n414 = while "Control_Loops" {
    tunnel: w3 -> [w772]
    tunnel: [w770] -> _
    tunnel: [TRUE] -> _
    i -> [w773]
    stop <- w770 stop-if-true
    n415 = call "MM_Module_Control.vi"("MM_Module_Ctrlr_Mode"=MM_Module_Control_Mode."Get", "Module Name"="Control_Loops") -> ("MM_Module_Action Out"=w774:T35)  [unwired: 6 in, 3 out]
    n416 = case shown="\"Idle\", Default" w774 {
      tunnel: w773 -> [_ _ _]
      tunnel: w772 -> [_ w776 _]
      tunnel: [_ _ TRUE] -> w770
      frame "Idle", Default {
        n417 = call "Wait with Error Clusters.vi"("Wait (mS)"=u32 100 ("Milliseconds to Wait (500)")) -> ()  [unwired: 14 in, 1 out]
      }
      frame "Start" {
        n418 = call "00_MOD_Control_Loops.vi"("Main Config File Refnum"=w776) -> ()  [unwired: 10 in, 1 out]
      }
      frame "Exit" {
      }
    }
  }
  n419 = while "Logging" {
    tunnel: w3 -> [w782]
    tunnel: [w780] -> _
    tunnel: [TRUE] -> _
    i -> [w783]
    stop <- w780 stop-if-true
    n420 = call "MM_Module_Control.vi"("MM_Module_Ctrlr_Mode"=MM_Module_Control_Mode."Get", "Module Name"="Logging") -> ("MM_Module_Action Out"=w784:T35)  [unwired: 6 in, 3 out]
    n421 = case shown="\"Start\"" w784 {
      tunnel: w783 -> [_ _ _]
      tunnel: w782 -> [_ w786 _]
      tunnel: [_ _ TRUE] -> w780
      frame "Idle", Default {
        n422 = call "Wait with Error Clusters.vi"("Wait (mS)"=u32 100 ("Milliseconds to Wait (500)")) -> ()  [unwired: 14 in, 1 out]
      }
      frame "Start" {
        n423 = call "Get Main Log Path and Name from Config.vi"("Main Config File Refnum"=w786) -> ("LogBaseName"=w787:string, "LogBasePath"=w788:path)  [unwired: 8 in, 1 out]
        n424 = call "GLOG_Logging Manager.vi"("LogBaseName"=w787, "LogBasePath"=w788) -> ()  [unwired: 10 in]
      }
      frame "Exit" {
      }
    }
  }
  n425 = while "Spare" {
    tunnel: w3 -> [w793]
    tunnel: [w791] -> _
    tunnel: [TRUE] -> _
    i -> [w794]
    stop <- w791 stop-if-true
    n426 = call "MM_Module_Control.vi"("Module Name"="Spare") -> ("MM_Module_Action Out"=w795:T35)  [unwired: 7 in, 3 out]
    n427 = case shown="\"Exit\"" w795 {
      tunnel: w794 -> [_ _ _]
      tunnel: w793 -> [_ _ _]
      tunnel: [_ _ TRUE] -> w791
      frame "Idle", Default {
        n428 = call "Wait with Error Clusters.vi"("Wait (mS)"=u32 100 ("Milliseconds to Wait (500)")) -> ()  [unwired: 14 in, 1 out]
      }
      frame "Start" {
        n429 = call "Wait with Error Clusters.vi"("Wait (mS)"=u32 100 ("Milliseconds to Wait (500)")) -> ()  [unwired: 14 in, 1 out]
      }
      frame "Exit" {
      }
    }
  }
  n430 = flat-sequence {
    tunnel: w9 -> [w799]
    tunnel: w2 -> [w800]
    frame #0 {
      n431 = Release Queue(queue=w800) -> ()  [unwired: 2 in, 3 out]
      n432 = call <vilib>:"Simple Error Handler.vi"("error in (no error)"=w799) -> ()  [unwired: 4 in, 5 out]
      n433 = flat-sequence {
        frame #0 {
          n434 = Wait (ms)(milliseconds to wait=u32 2000) -> ()  [unwired: 1 out]
        }
        frame #1 {
          n435 = call "GLOG_Logger_Methods.vi"("Logger Method"=T36."SHUTDOWN") -> ()  [unwired: 9 in, 2 out]
        }
      }
    }
    frame #1 {
      n436 = disable-structure shown="RUN_TIME_ENGINE==True, default" {
        disable-tunnel: [TRUE TRUE] -> w803
        frame condition #0 {
          n437 = Quit LabVIEW() -> ()  [unwired: 1 in]
        }
        frame condition #1 (active) {
        }
      }
      n438 = case shown="True" w803 {
        frame False {
        }
        frame True {
          n439 = property class="VI"("Front Panel.Open"=FALSE) -> (error out=w806:errorcluster)  [unwired: 2 in, 1 out]
          n440 = stacked-sequence {
            tunnel: w806 -> [_]
            frame #0 {
            }
          }
        }
      }
    }
  }
